vi "Argos_K_4.0 (SUPTNIK Customized Edition).vi"(0 "PID 1 COM":refnum<visa-resource-name>="COM1", 1 "Setpoint\n START":bool, 2 "Write to File":bool, 3 "SP 1 input (°C)":dbl=20.0 min=0.0 max=1300.0, 4 "Intervall (s)":u32=1 max=600, 5 "Write/\nRead":bool=TRUE, 6 "Delay (ms)":u32=500 min=100 max=600000, 7 "Auto Tune":bool, 9 "Standby":bool, 11 "Reset\nSTOPP":bool, 12 "ON":bool=TRUE caption="OFF", 13 "Get Values":bool, 15 "File Path":path) -> (8 "(°C)":dbl format="%#.3f", 14 "SP 1 is (°C)":dbl)   [LabVIEW 2013]
doc: "1. Verwendung\n\nDas Programm dient der Steuerung und Abfrage des Thermocontrollers I3252 und dem Auslesen von zwei VC 840 Messgeräten und einem Druckmessgerät Pfeiffer Single Gauge. \nDie Messgeräte werden Standardmäßig ausgelesen und erst nach Betätigung des Schalters \"Write to File\" in einer Textdatei abgespeichert. Das Eingabefeld \"Intervall\" legt den Abstand der Messpunkte fest.\nDer Setpoint für den Thermocontroller wird erst nach Betätigung des Tasters \"Setpoint START\" übernommen und angesteuert. Er wird ind den EEPROM des Gerätes geschrieben. Die Regelung kann mit Hilfe des Schalters \"Standby\" unterbrochen werden. Durch den Taster \"Reset STOPP\" kann der Setpoint aus dem EEPROM gelöscht werden.\nDie Eingabeflächen \"Constant\" und \"Thickness\" dienen der Berechnung des spezifischen Widerstands.\nDie Eingabeflächen \"User\" und \"Sample\" werden in den Header der Textdatei übernommen.\nDer Indikator \"File Path\" zeigt den aktuellen Speicherort der Textdatei an. Dieser wird nach ausschalten des Schalters \"Write to File\" gelöscht. Bei erneuten Schreiben muss ein neuer Speicherort gewählt werden. Bei Wahl desselben Speicherorts werden sämtliche bereits gespeicherte Daten gelöscht.\n\n\n2. Erläuterungen zum Blockdiagramm\n2.1 äußere Sequenz\nDie äußerte Sequenz besteht aus fünf Frames. Der erste dient der Initialisierung der Ports. Der zweite dient als Verzögerung um dem Programm genug Zeit zu geben die Ports zu öffnen. Jedoch senden die beiden VC 840 bereits Informationen an den Computer die in einem Puffer zwischengespeichert werden. Im dritten Frame wird dieser Puffer geleert. Somit kommt es zu keinem Framing Error. Desweiteren wird in diesem Frame die Startzeit der Messungen genommen. Im vierten Frame wird die eigentliche Messung und Verarbeitung der Daten durchgeführt. Die while-Schleife wird nur durch Auftreten eines Fehlers oder durch Betätigung des Stopbuttons auf dem Front Panel in der oberen linken Ecke unterbrochen. Im fünften und letzten Frame werden die Ports wieder geschlossen und beim Auftreten eines Fehlers wird das Programm automatisch gestoppt. Falls kein Fehler auftritt wird die Sequenz von vorne abgearbeitet.\n\n2.2 while-Schleife und innere Sequenz\n2.2.1 \"Event Structure\"\n2.2.1.1 Allgemein\nDer erste Frame beinhaltet ein \"Event Structure\". Dieser reagiert auf insgesamt elf verschiedene Ereignisse. Falls keines dieser Ereignisse auftreten sollte, warte die Struktur eine Millisekunde bevor die \"Event Structure\" verlassen wird. Die übrigen Ereignisse treten ein, wenn der entsprechende Kontroller eine Werteänderung erfährt.\n\n2.2.1.2 Event: Setpoint\nDieser Case besteht von außen nach innen aus einer Stacked Sequence, einer for-Loop und einer Flat Sequence die wiederum zwei \"Case Structures\" enthält. Als erstes wird bei dem Schalter \"Setpoint START\" der Blinkmodus aktiviert und bei dem Schalter \"Read Temperature\" deaktiviert. Danach folgt das eigentliche setzen des Temperatursollwerts. In der ersten Iteration wird dem Controller I3252 ein Schreibbefehl gesendet. Theoretisch kann der Setpoint in den RAM oder in den EEPROM geschrieben werden. Diese Auswahl erfolgt mit Hilfe des Schalters \"RAM\". Da das Schreiben in den RAM -Speicher aber aus diversen Gründen nicht erwünscht ist, wurde es nicht implementiert. Eine nachträgliche Implementierung ist aber leicht möglich, in dem die untere String-Konstante \"*P012\" durch \"*W012\" ersetzt wird. An diesem Befehl wird eine fünfstellige Hexadezimalzahl angehängt, die den Sollwert wiedergibt. Der Sollwert wird vorher mit zehn multipliziert, da das Komma standardmäßig nach der ersten Ziffer festgesetzt wurde (Bsp.: 800 wird gesendet um 80 einzustellen). Dieser Befehlsstrang wird an das Gerät mittels des SubVIs \"Comm_Interface\", auf welches später noch näher eingegangen wird, weitergegeben. Der durch das Gerät zurückgegebene String wird nicht verarbeitet.\nDie zweite Iteration dient dem Auslesen des eingestellten Sollwertes. Wahlweise kann der RAM- oder der EEPROM-Speicher ausgelesen werden. Die eigentliche Verarbeitung des Ausgabestrings erfolgt durch das SubVI \"Edit Setpoint\".\nDie Implementierung zur Einstellung des zweiten Setpoints erfolgt durch kopieren der ersten beiden Fälle und ersetzen der \"1\" im Befehf durch eine \"2\" (Bsp.: \"*P012\" zu \"*P022\"). Es darf aber nicht vergessen werden, dass dann ebenfalls die Anzahl der Iterationen angepasst werden muss.\nAls letztes wird der Blinkmodus des Schalters \"Setpoint START\" wieder deaktiviert.\n\n2.2.1.3 Event: Standby\nDieses Ereignis aktiviert bzw. deaktiviert als erstes den Blinckmodus des entsprechenden Schalters und sendet danach den Befehl zum aktivieren (\"*D03\") oder zum deaktivieren (\"*E03\") des Standbymodus an den Thermocontroller.\n\n2.2.1.4 Event: Set Command \nDer in das Feld \"Command shall be\" eingegebene Befehl wird an den Thermocontroller übermittlet. Die korrekte Form des Befehls ist im \"Communication Manuel\" nachzuschlagen. Das \"*\"-Zeichen wurde allerdings schon implementiert und muss somit nicht mit eingegeben werden.\n\n2.2.1.5 Event: Reset\nIn der ersten Iteration wird der Reset-Befehl an den Thermocontroller gesendet. In Folge wird der gesamte EEPROM-Speicher gelöscht. Deshalb wird in der zweiten Iteration der Setpoint aktualisiert. Dieser Befehl hat keinen Einfluss auf den RAM-Speicher. Die anschließende Wartezeit ist auf vier Sekunden festgesetzt und wurde empirisch ermittelt. Diese Zeit benötigt das Gerät um den Reset durchzuführen und für die Kommunikation wieder zur Verfügung zu stehen.\n\n2.2.1.6 Event: Auto Tune\nEs ist festgeschrieben, dass der Setpoint für die \"Auto Tune\"-Funktion wenigstens 20°C über der aktuellen Temperatur liegt. Deshalb wird zunächst der aktuelle Temperaturwert ausgelesen. Im zweiten Schritt werden zu diesem Wert zwanzig addiert und der Setpoint wird in den RAM-Speicher geschrieben. Das Schreiben in diesen Speicher ist nötig, da die \"Auto Tune\"-Funktion\" erst nach einem Reset startet. Im dritten Schritt wird der eigentliche Befehl für den \"Auto Tune\" gesendet (siehe dazu \"Communication Manuel\" S.27). Als vierte und letzte Iteration der for-Schleife folgt der bereits erwähnte Reset-Befehl. Der Temperatursollwert, der im RAM-Speicher eingetragen ist, muss zum Schluss wieder auf 0°C gesetzt werden. Die Zeit für die Ausführung des \"Auto Tune\"-Befehls wurde empirisch ermittelt und 45 s festgesetzt.\n\n2.2.1.7 Event: Write LOW/HI\nDieses Ereignis setzt die am Analogausgang anliegende Spannung fest. Normalerweise beträgt dieser Spannungswert 0-10 V. Das angeschlossene Netzteil verträgt aber maximal nur 2,3 V. Aus diesem Grund wird der \"%HIGH\" auf 23 gesetzt. Somit beträgt die maximal anliegende Spannung nur noch 23% von der maximal möglichen, d.h 2,3V. Ein niedrigerer Wert ist jederzeit möglich, genauso wie ein höherer für den Parameter \"%LOW\". Diese werden zunächst nacheinander in den RAM-Speicher geschrieben und anschließend wieder ausgelesen.\n\n2.2.1.8 Event: Set PID\nDie Werte für den PID-Regler können sowohl mit Hilfe der \"Auto Tune\"-Funktion, als auch manuell eingestellt werden. Es wird wiederum zwischen dem Schreiben in den RAM- und dem EEPROM-Speicher unterschieden. Zunächst werden die Werte für \"P\", \"I\" und \"D\", in dieser Reihenfolge, gesetzt und danach die aktuellen Werte ausgelesen.\n\n2.2.1.9 Event: Get Values\nDieses Ereignis hat zur Folge, dass die Werte für \"P\", \"I\", \"D\", \"%LOW\", \"%HIGH\" und des Setpoints wahlweise aus dem RAM- oder EEPROM-Speicher gelesen werden. Die aktuellen Werte werden nicht nur in die entsprechenden Anzeigefelder übernommen, sondern auch in die entsprechenden Eingabefelder, mit Ausnahme des Temperatursollwerts. \n\n2.2.1.10 Event: RAM\nPrinzipiell kann zwischen dem Schreiben in den RAM- oder EEPROM-Speicher des Thermocontrollers gewählt werden. Die entsprechende Schalterposition auf dem Frontpanel zeigt den aktuell verwendeten Speicher an. Die Anzeigewerte werden bei jedem Umschalten aktualisiert und sind im entsprechenden Speicher eingetragen. Die Implementierung ist identisch mit der des Ereignisses \"Get Values\". Es gilt zu beachten, dass die Werte für \"%LOW\" und \"%HIGH\" nur in den RAM-Speicher geschrieben werden können und somit auch nur aus diesem ausgelesen werden können.\n\n2.2.1.11 Event: Set Gauge to Zero\nMit Hilfe der SubVIs \"Get Pressure\" und \"Offset Display\" werden die Werte für den alten und den neuen Offset und der durch den zweiten Drucksensor ermittelt Druck ermittelt. \n\n2.2.1.12 Event: Write to File\nSollte der Schalter \"Write to File\" aktiviert werden, d.h. Schalterposition oben, so wird zunächst durch das SubVI \"Header\" ein Header für die unter \"File Path\" definierte Datei angelegt. Alle Werte, die bereits in der entsprechenden Datei stehen, werden dabei gelöscht.\n\n2.2.2 \"Timed Structures\"\nIm dritten Frame der inneren Sequenz werden die Werte für Zeitpunkt, Temperatur, Spannung, Strom und Druck ermittelt. Damit die Werte zum gleichen Zeitpunkt aufgenommen werden, werden \"Timed Sequences\" eingesetzt. Mit dem entsprechenden Schalter auf dem Front Panel unter dem Tab \"Settings\" kann gewählt werden, ob das entsprechende Gerät ausgelesen werden soll oder nicht. Die einzelnen Sequenzen werden parallel abgearbeitet, womit die Prozesszeit von diesem Frame durch der zeitintensivsten Sequenz abhängt. Dies ist in aller Regel das Auslesen der Temperatur, da ein \"Delay\" von 500 ms oder größer benötigt wird, um den Controller ordentlich ansprechen zu können.\nDie Systemzeit wird durch das SubVI \"System Time in Seconds\" in Sekunden umgerechnet und der in dem Parameter \"Starttime\" gespeicherte Wert wird abgezogen. Somit werden die Sekunden seit dem Start des Programms gezählt.\n\n2.2.3 restlichen Frames\nIm zweiten Frame wird das Intervall zwischen den einzelnen Messwerten festgelegt. Dabei wird der Wert des Parameters \"Delay\" abgezogen. Dieser Wert beträgt im Normalfall 500 ms und ist somit nicht vernachlääsigbar.\nDer Vierte Frame beinhaltet die Umrechnung des Temperatur-Strings in einen Temperaturwert durch das SubVI \"Edit Tmperature\", die Berechnung des spezifischen Widerstands durch das SubVI \"Resistivity Calculation\" und die Überprüfung des Druckwerts. Auch werden die neu gewonnen Werte in das entsprechende Shift-Register übernommen. Falls der Druckwert einen in dem Parameter \"Pressure Limit (mbar)\" festgelegten Grenzwert überschreiten sollte, wird der Thermocontroller automatisch in den Standby-Modus versetzt. Des Weiteren wird der Schalter \"Standby\" solange gesperrt, wie der Druck oberhalb des Grenzwertes liegt. Wenn der Druck wieder unter den Grenzwert gesunken ist, wird der Standby-Befehl nicht automatisch aufgehoben, sondern muss vom Benutzer durch Betätigung des entsprechenden Schalters gegeben werden.\nIm fünften Frame werden die Diagramme erstellt. Dabei wird jedes Mal von neuem das gesamte Shift-Register als Graph dargestellt. Weiterhin werden die Messwerte in ein 1D-Array geschrieben.\nDer sechste und letzte Frame beinhaltet den eigentlich Schreibvorgang der Messwerte in eine Textdatei und die Überprüfung ob ein Fehler vorliegt.\n\n2.3 SubVIs\n2.3.1 Allgemein\nDie SubVIs für die Messgeräte VC840 und das Druckmessgerät wurden aus anderen Quellen übernommen. \n\n2.3.2 \"Header\"\nIn den Header wird zunächst das aktuelle Datum und die aktuelle Zeit übernommen. Die ausgewählte Datei wird dabei überschrieben. Danach wird der Name des Benutzers und der Probe übernommen. Zum Schluss werden die Einheiten in einer Reihe, durch einen Tabulator getrennt, in den Header geschrieben.\n\n2.3.3 \"I3252 Comm Interface\"\nDieses VI stellt die Kommunikation mit dem Thermocontroller her und gibt den Ausgabe-String zurück.\n\n2.3.4 \"I3252 Edit Setpoint\"\nIm Ausgabe-String vom Thermocontroller ist an der vierten Stelle die Stelle des Dezimalpunktes verschlüsselt. Dieses Hexadezimalzahl wird herausgefiltert und an ein \"ENUM Controller\" übergeben. Dieser weist der Hexadezimalzahl eine Nummer zu, mit welcher ein Wert aus einem Array entnommen wird. Dieser Wert dient als Quotient. Der tatsächliche Wert kann somit errechnet werden.\n\n2.3.5 \"I3252 Edit Temperature\"\nDer Temperatur-String, der vom Thermocontroller zurückgegeben wird, wird in eine Dezimalzahl umgewandelt. Manchmal kommt es aus zu Dropouts, die durch dieses Programm herausgefiltert werden. Der letzte Wert wird dabei in einer \"Feedback Node\" gehalten unter der Annahme, dass sich der Temperaturwert nicht sprunghaft ändert.\n\n2.3.6 \"Resistivity Calculation\"\nDer spezifische Widerstand wird nach folgender Formel ausgerechnet. Dabei entspricht t der Dicke der Probe und C ist eine Konstante.\nrho=C*pi*t*U/(ln( 2)*I)\n\n2.3.7 \"System Time in Seconds\"\nZunächst wird die aktuelle Systemzeit ausgelesen. Danach wird diese in Stunden, Minuten und Sekunden aufgeteilt, alles in Sekunden umgerechnet und letztendlich addiert."
uses:
  <vilib>/Platform/TimedLoop/XDataNode/timing_clust.ctl
  <vilib>/Platform/TimedLoop/XDataNode/nitl_modes.ctl
  <vilib>/Platform/TimedLoop/XDataNode/wakeup.ctl
  <vilib>/Instr/_visa.llb/VISA Configure Serial Port (Instr).vi
  <vilib>/Platform/TimedLoop/scheduler/LVUserAPI/_suppVIs/Create_1kHz_TSource.vi
  <vilib>/Utility/file.llb/Write To Spreadsheet File (DBL).vi
  <vilib>/Platform/TimedLoop/XDataNode/XDataNode.xnode
  <vilib>/Platform/TimedLoop/XDataNode/XDNodeRunTimeDep.lvlib
  Argos0v7/Dependencies/Pfeiffer TPG261+262 Single+Dual Gauge/Dual Gauge.lvlib
panel:
  out "appended array":dbl[](array[numeric])
  in  "Tab Control":T1(tab)
  out "Get Actual Set Point":dbl
  in  "Get SetPoint":bool
  in  "Setpoint":dbl=10.0
  in  "Minutes":dbl
  in  "Hours":dbl
  in  "Soak Minutes":dbl=1.0
  in  "Soak Hours":dbl
  in  "Ramp":bool
  in  "Sample":string
  in  "User":string
  out "Thermocouple (Sample holder 1)":cluster{dbl[], dbl[]}(graph)
  out "current time (s)":dbl
  out "data logger intervall (s)":dbl
  out "loop time (s)":dbl
  in  "stop":bool
  out "TPG 1":cluster{dbl[], dbl[]}[](graph)
  out "Pressure Baratron 2":dbl format="%#_4e"
  out "Pressure FullRange 2":dbl format="%#_3e"
  out "Pressure OpenPort":cluster{dbl[], dbl[]}(graph)
  out "Pressure OpenPort2":dbl caption="current"
  in  "PID 2 COM":refnum<visa-resource-name>="COM8"
  in  "Baud Rate 2":u32=9600
  in  "Data Bits 2":u16=7 min=5 max=8 step=1
  in  "Parity 2":u16(ring)=1 items=["None", "Odd", "Even", "Mark", "Space"]
  in  "Stop Bits 2":u16(ring)=10 items=["1.0"=10, "1.5"=15, "2.0"=20]
  in  "Flow Control 2":u16(ring) items=["None"=0, "XON/XOFF"=1, "RTS/CTS"=2, "DTR/DSR"=4]
  in  "Delay (ms) 2":u32=500 min=100 max=600000
  in  "Write/\nRead 2":bool=TRUE
  out "status 2":bool caption="Status"
  out "code 2":i32 caption="Code"
  out "code":i32 caption="Code"
  out "status":bool caption="Status"
  in  "Set Gauge to Zero":bool
  out "Status Gauge 1#2":i32(ring) items=["data OK", "underrange", "overrange", "sensor error", "sensor off", "no sensor", "ID error"]
  out "Pressure Gauge 1#2":dbl format="%.3e"
  out "Pressure Gauge 1#1":dbl format="%.3e"
  out "Status Gauge 1#1":i32(ring) items=["data OK", "underrange", "overrange", "sensor error", "sensor off", "no sensor", "ID error"]
  in  "TPG 1 COM":refnum<visa-resource-name>="COM5"
  in  "Pressure Limit (mbar)":dbl=1.0 min=0.0 max=1100.0
  out "Current Offset (mbar)":dbl
  in  "ON (TPG 2)":bool caption="OFF"
  in  "ON (TPG 1)":bool=TRUE caption="OFF"
  in  "ON":bool caption="OFF"
  in  "VC 840 2":refnum<visa-resource-name>="COM8"
  out "Reading 2":dbl format="%_4f"
  out "Mode 2":enum16{"?", "Diode", "Beep", "DC", "AC"}(ring)
  out "Unit 2":string
  in  "VC 840 1":refnum<visa-resource-name>="COM8"
  out "Reading 1":dbl format="%_4f"
  out "Mode 1":enum16{"?", "Diode", "Beep", "DC", "AC"}(ring)
  out "Unit 1":string
  out "Status 1":T2
  out "Status 2":T2
  in  "ON":bool caption="OFF"
  out "% HIGH Istwert":u32
  out "% LOW Istwert":u32
  in  "% High Sollwert":u32=23 max=24
  in  "% LOW Sollwert":u32 max=25
  in  "RAM":bool=TRUE caption="EEPROM"
  out "D (Rate) IstWert":u32
  out "I ( Reset1) Istwert":u32
  out "P (PB1) Istwert":u32 caption="actual value"
  in  "D (Rate) Sollwert":u32 max=3999
  in  "I ( Reset1) Sollwert":u32 max=3999
  in  "P (PB1) Sollwert":u32 caption="set value" max=9999
  in  "Set Command":bool
  in  "Set PID":bool
  in  "Write LOW/HI":bool
  in  "Flow Control":u16(ring) items=["None"=0, "XON/XOFF"=1, "RTS/CTS"=2, "DTR/DSR"=4]
  in  "Stop Bits":u16(ring)=10 items=["1.0"=10, "1.5"=15, "2.0"=20]
  in  "Parity":u16(ring)=1 items=["None", "Odd", "Even", "Mark", "Space"]
  in  "Data Bits":u16=7 min=5 max=8 step=1
  in  "Baud Rate":u32=9600
  out "Command output":string
  in  "Command input":string
  in  "TPG 2 COM":refnum<visa-resource-name>="COM8"
  out "Pressure Gauge 2#2":dbl format="%.3e"
  out "Pressure Gauge 2#1":dbl format="%.3e"
  out "Status Gauge 2#2":i32(ring) items=["data OK", "underrange", "overrange", "sensor error", "sensor off", "no sensor", "ID error"]
  out "Status Gauge 2#1":i32(ring) items=["data OK", "underrange", "overrange", "sensor error", "sensor off", "no sensor", "ID error"]
  out "Current":cluster{dbl[], dbl[]}(graph)
  out "Voltage":cluster{dbl[], dbl[]}(graph)
  out "Voltage (V)":dbl format="%.4e"
  out "Current (A)":dbl format="%.4e"
  out "Resistivity":cluster{dbl[], dbl[]}(graph)
  out "Resistivity (Ohm*cm)":dbl format="%.3e"
  out "Pirani (VVP1 Scroll)":cluster{dbl[], dbl[]}(graph)
  in  "4PP constant":dbl min=0.0 max=5.0
  in  "Thickness (nm)":dbl min=0.0
  out "Pressure Pirani 2":dbl format="%#_3e"
  # "set \nvalue"
  # "actual \nvalue"
  # "T (°C)"
  # "Ramp And Soak Toolkit"
  # "Ramp"
  # "Soak"
  # "mbar"
  # "mbar"
  # "mbar"
  # "Pressure Measurement \n(Pfeiffer TPG261)"
  # "PID Controller (Omega Newport i3252)"
  # "PID Controller (Omega Newport i3252)"
  # "limit (mbar)"
  # "Multimeter\n#1 (VC 840)"
  # "Multimeter\n#2 (VC 840)"
  # "P"
  # "I"
  # "D"
  # "% Low"
  # "% High"
  # "mbar"
  # "Authors:  Daniel Schuster (sir-dan@web.de)\n                 Steffen Cornelius (s.cornelius@hzdr.de)\n                 Nico Spahn (x)\n\n                 premade SubVIs for readout of Pfeiffer gauge and VC840 Multimeters were used\n                 SubVI \"I3252_Comm_Interface\" is based on a modified Labview example\n\nRelease:  v1.0    \n\nVersion History:\n\nv1.1  -    28.06.2011\n             - Format des Files geändert von %.3f auf %g\n             - maximale Eingabewerte für PID begrenzt\nv1.2  -    12.07.2011\n             - Anzeige p,rho, U, V auf Scientific geändert\n             - y-Achse p,rho auf Log geändert\n             - numerische Zeitanzeige hinzugefügt\n             - 4PP Constant: pi/ln(2)=4,532 set as the default value\nv1.3  -    25.07.2011\n             - Zeitvariable auf EXT geändert, um Sprünge in Diagrammen loszuwerden\nv1.4  -   27.07.2011\n             - ALLE Variablen auf DBL zurückgesetzt wegen Formatierungsproblem im File\n             - Zeitberechnung neu gemacht (Tick count differenzen) -> Zeitsprünge korrigiert ?\n             - Delay/Intervall überarbeitet\nv1.5  -   05.12.2012\n                - Austausch der alten Pfeifer SubvIs durch neue -> nun alle 4 Kanäle des DualGauge\n                                                                                                         Controllers gleichzeitig auslesbar\n                - neue Pfeiffer SubVIs verwendet in Druckwertauslesung und Offset Berechnung des Baratron\n                  Druckes (COM5 Sensor1)\n                - Neuarragement des GUI -> FullRange und Baratron neben Temperatur auf Haupseite zu sehen\n                                                                   Pirani und OpenPort auf Meas.2 zu sehen\n                                                                   Diagnose Seite umfasst nun auch Widerstandsdiagramm\n                - Änderungen der Settingseite -> nun alle 4 Drucksensoren mit aktuellem Messwert und Gerätestatus\n                                                                           zu sehen\n                - The readout of the PID-Temperature Controller and the VC840 Multimeters was not modified\nv1.73  -  18.10.2013\n                - Layout Änderungen\nv.1.8   -  19.01.2014\n                - Änderung Layout Settings Tab\n                - Trennung der beiden TPG Dual Gauge Controls\n                -"
  # "Version 1.73    - last change 18.10.2013"
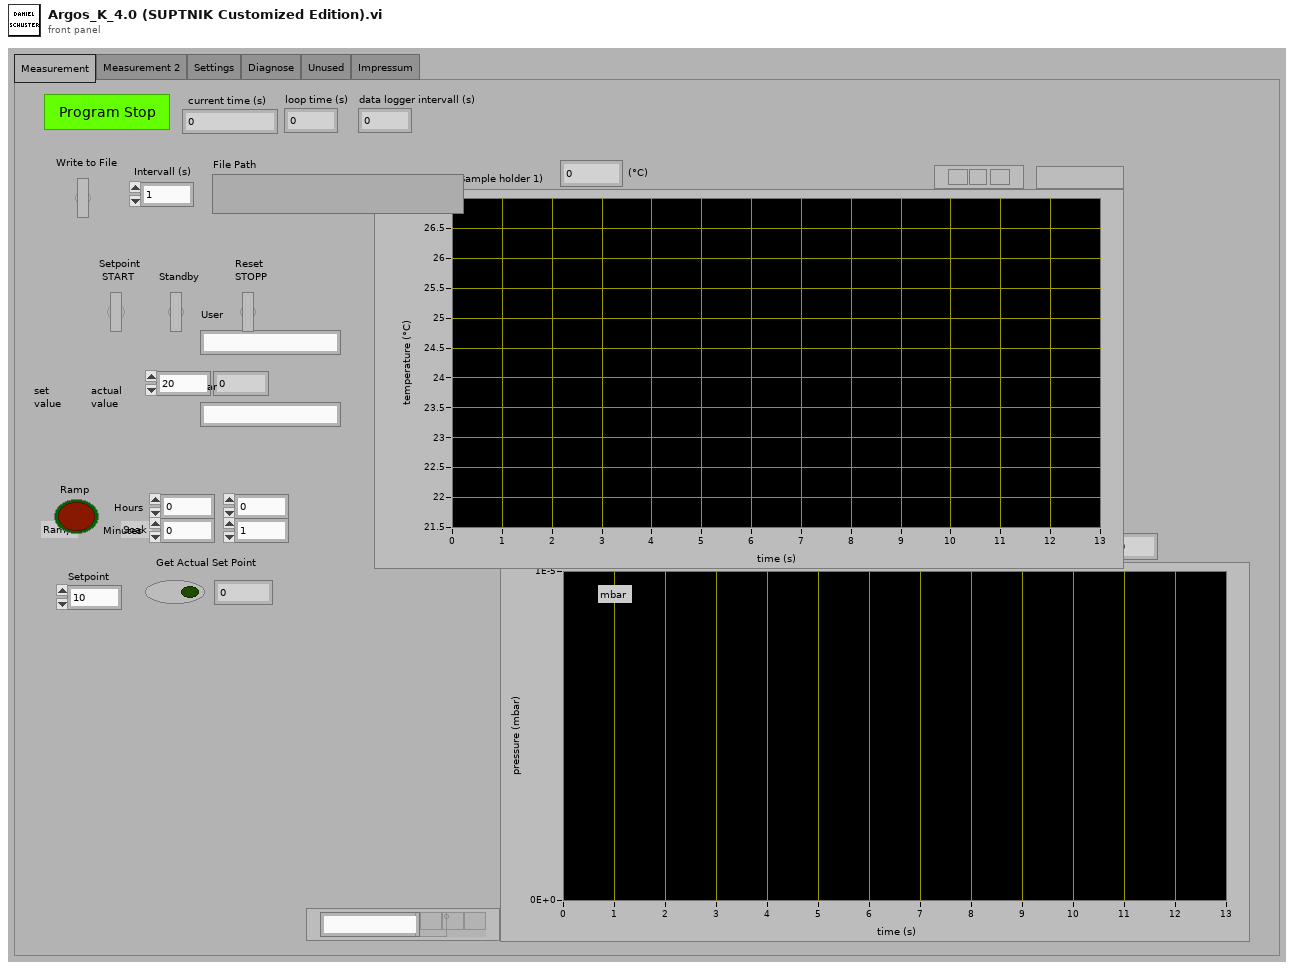
[diagram p1: front panel]
types:
  T1 = enum32{"Measurement", "Measurement 2", "Settings", "Diagnose", "Unused", "Impressum"}
  T2 = cluster{"Low Bat":bool, "Auto":bool, "Delta":bool, "Hold":bool, "RS232":bool}
  T3 = typedef "XDNodeRunTimeDep.lvlib/timing_clust.ctl" = cluster{"Expected End [f-1]":u64, "Actual End [f-1]":u64, "Finished Late? [f-1]":bool, "Expected End [i-1]":u64, "Actual End [i-1]":u64, "Finished Late? [i-1]":bool, "Expected Start [i]":u64, "Actual Start [i]":u64, "Expected Start [f]":u64, "Actual Start [f]":u64, "Source Name":string, "Structure Name":string, "Period":i64, "Deadline":i64, "Offset":i64, "Start":i64, "Priority":i32, "Timeout":i32, "Mode":T4, "Wakeup Reason":T5, "Error":errorcluster, "Source Type":string, "Secondary Source Type":string, "Global End Time":u64, "Global Start Time":u64, "Frame Duration":u64, "Iteration Duration":u64, "Assigned CPU":i32, "I/O Scan Engine Mode":u32}
  T4 = typedef "XDNodeRunTimeDep.lvlib/nitl_modes.ctl" = enum32{"No Change", "Process missed periods, maintain original phase", "Discard missed periods, maintain original phase", "Process missed periods, ignore original phase", "Discard missed periods, ignore original phase"}
  T5 = typedef "XDNodeRunTimeDep.lvlib/wakeup.ctl" = enum32{"Normal", "Aborted", "Asynchronous wakeup", "Timing source error", "Timed loop error", "Timeout"}
  T6 = enum8{"Enabled", "Disabled", "Disabled and Grayed Out"}
  T7 = cluster{"VISA resource name out":refnum<visa-resource-name>, "error out":errorcluster, "Delay (ms)":u32, "Write/\nRead":bool}
  T8 = cluster{"VISA resource name out":refnum<visa-resource-name>, "error out":errorcluster, "Delay (ms) 2":u32, "Write/\nRead 2":bool}
  T9 = cluster{"TPG 2 COM":refnum<visa-resource-name>, "error out":errorcluster}
  T10 = cluster{"COM out":refnum<visa-resource-name>, "Cluster (Ausgang)":errorcluster}
  T11 = cluster{"Pressure Gauge#1":dbl, "Pressure Gauge#2":dbl}
  T12 = cluster{"TPG 1 COM":refnum<visa-resource-name>, "error out":errorcluster}
  T13 = cluster{"COM out":refnum<visa-resource-name>, "error out":errorcluster, "COM out":refnum<visa-resource-name>, "error out":errorcluster}
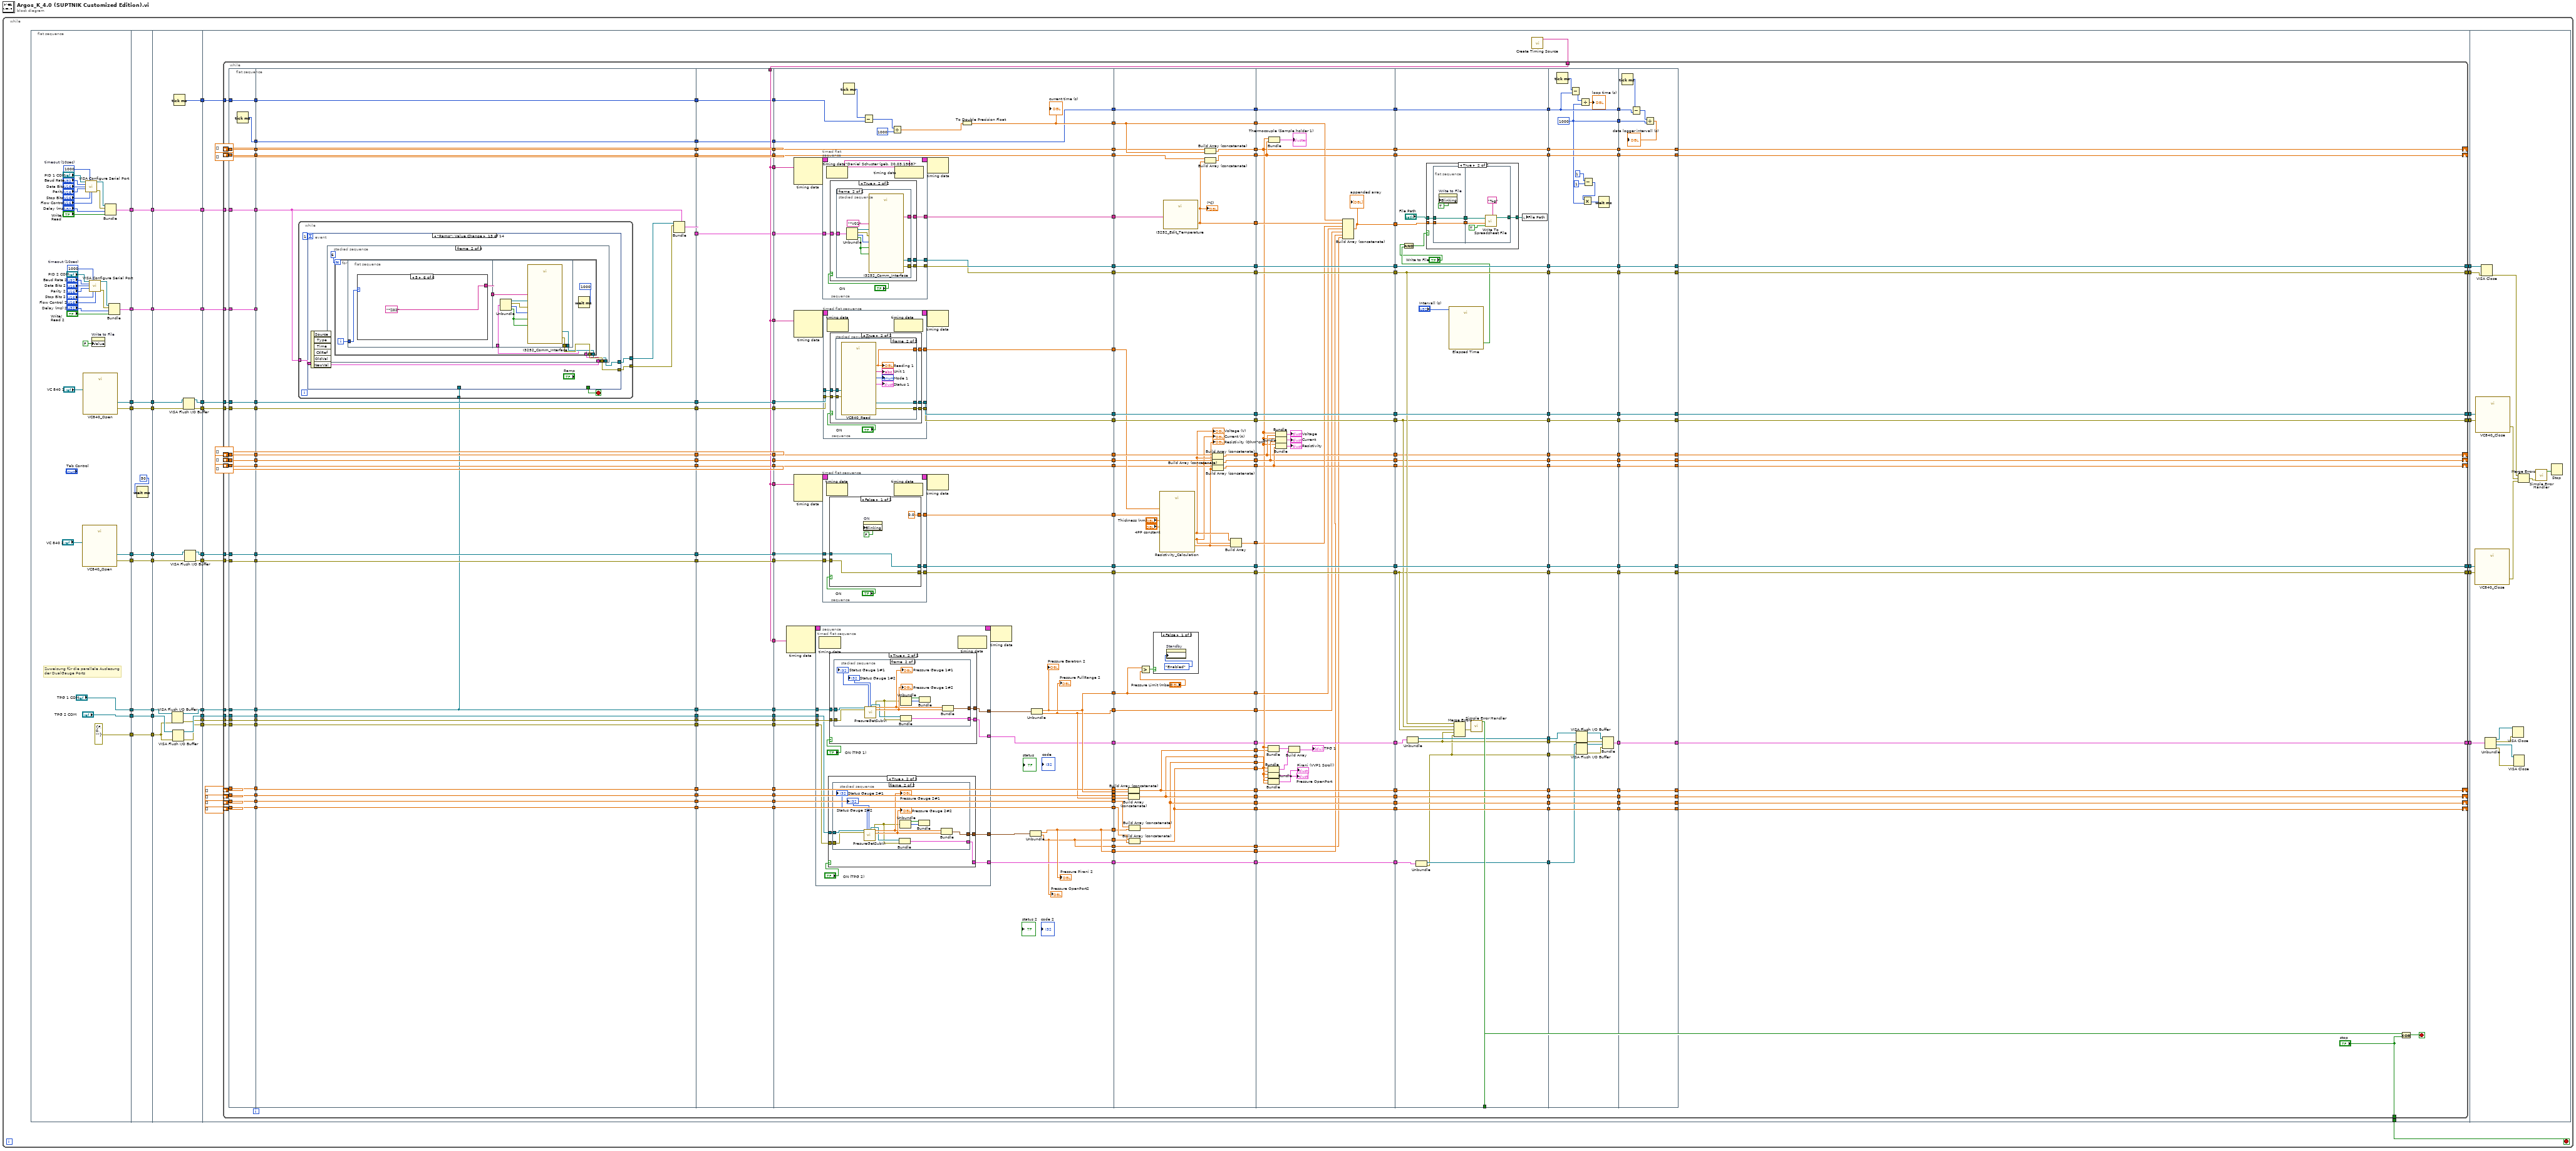
[diagram p0: block diagram]
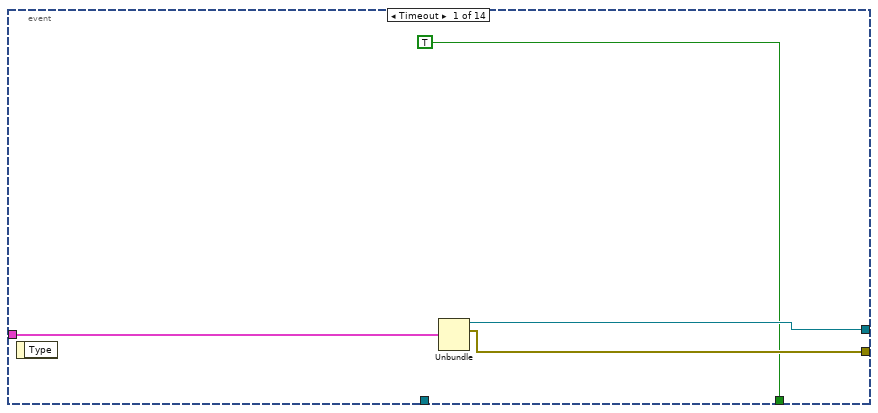
[diagram p2: hidden frame]
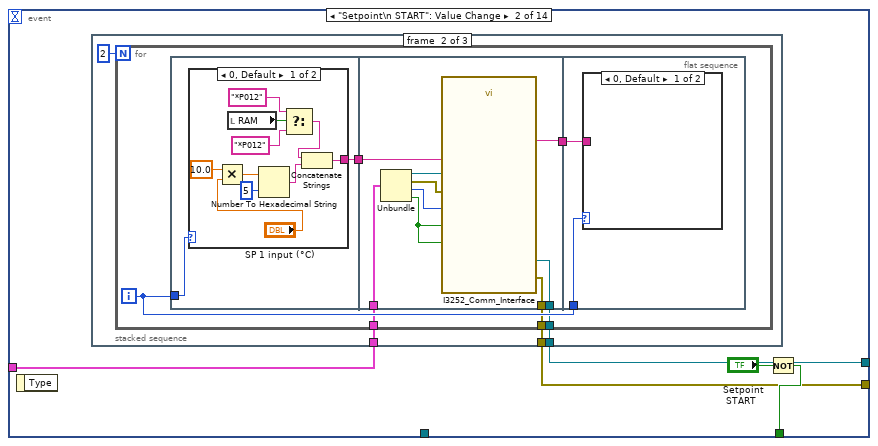
[diagram p3: hidden frame]
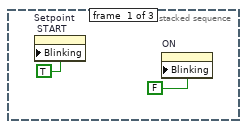
[diagram p4: hidden frame]
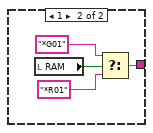
[diagram p5: hidden frame]
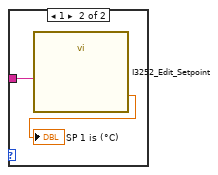
[diagram p6: hidden frame]
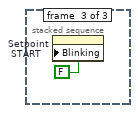
[diagram p7: hidden frame]
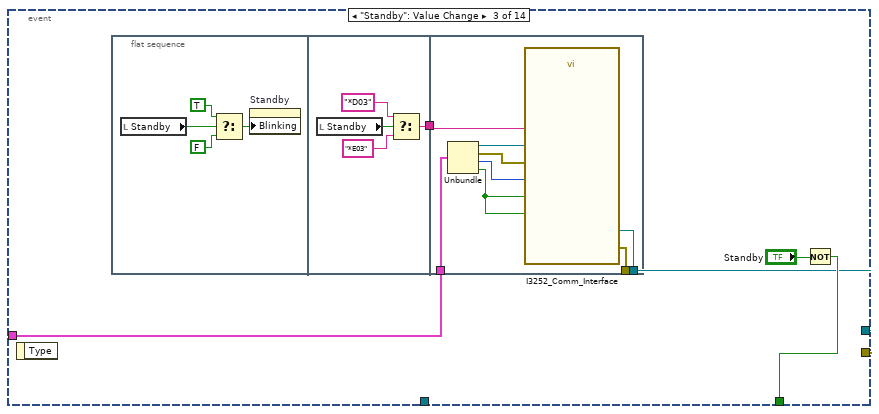
[diagram p8: hidden frame]
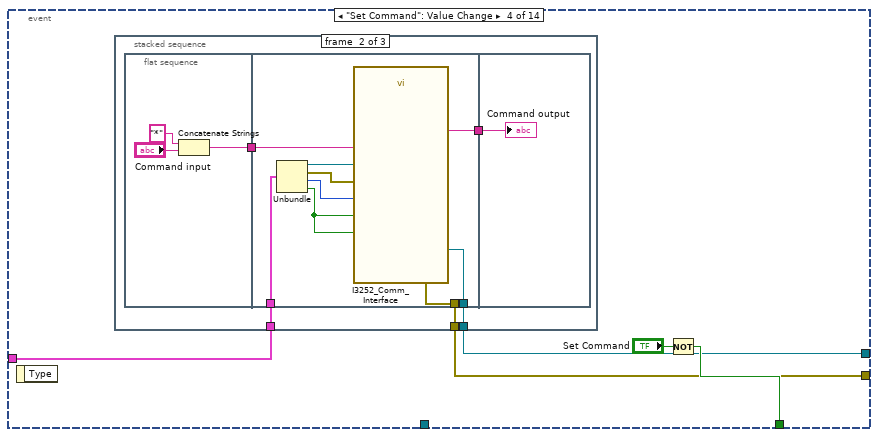
[diagram p9: hidden frame]
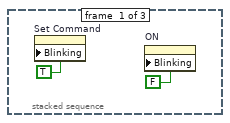
[diagram p10: hidden frame]
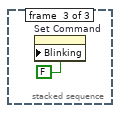
[diagram p11: hidden frame]
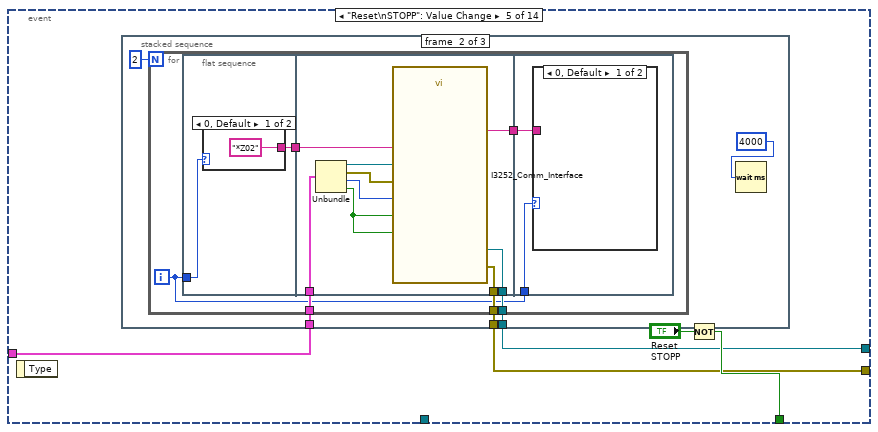
[diagram p12: hidden frame]
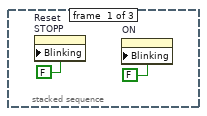
[diagram p13: hidden frame]
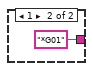
[diagram p14: hidden frame]
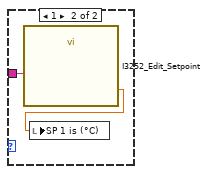
[diagram p15: hidden frame]
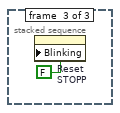
[diagram p16: hidden frame]
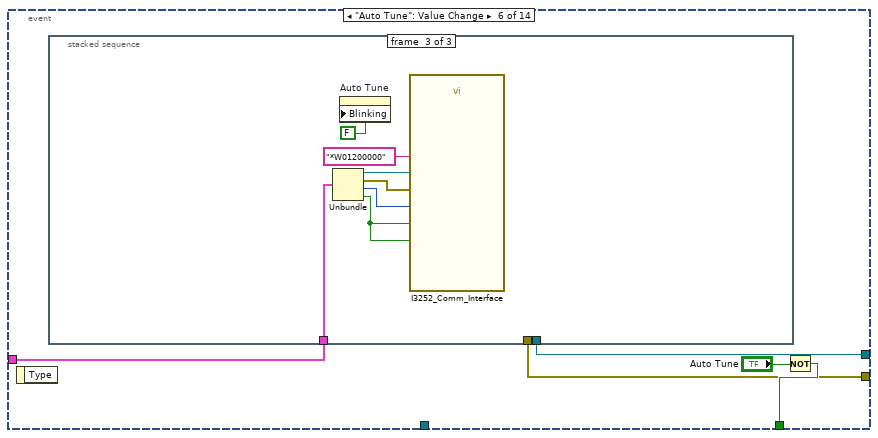
[diagram p17: hidden frame]
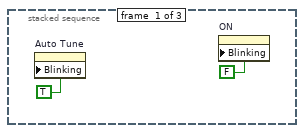
[diagram p18: hidden frame]
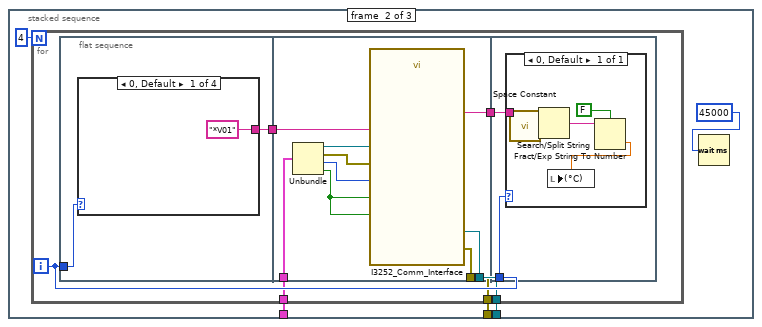
[diagram p19: hidden frame]
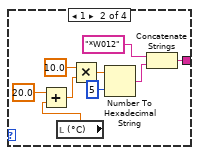
[diagram p20: hidden frame]
diagram:
  n1 = while {
    stop <- w9 stop-if-true
    n2 = flat-sequence {
      tunnel: [w70] -> w37
      tunnel: [w71] -> w36
      tunnel: [w56] -> w35
      tunnel: [w69] -> w34
      tunnel: [w68] -> w33
      tunnel: ["TPG 1 COM"] -> w32
      tunnel: ["TPG 2 COM"] -> w31
      tunnel: [errorcluster {"status"=FALSE, "code"=0, "source"=""} ("Fehler (Eingang)")] -> w6
      tunnel: [w39] -> w1
      tunnel: w37 -> [w81]
      tunnel: [w81] -> w30
      tunnel: w36 -> [w80]
      tunnel: [w80] -> w29
      tunnel: w35 -> [w79]
      tunnel: [w79] -> w28
      tunnel: w34 -> [w78]
      tunnel: [w78] -> w27
      tunnel: w33 -> [w77]
      tunnel: [w77] -> w26
      tunnel: [w75] -> w25
      tunnel: w32 -> [w75]
      tunnel: [w74] -> w24
      tunnel: w31 -> [w74]
      tunnel: [w73] -> w7
      tunnel: w6 -> [w73]
      tunnel: [w72] -> w2
      tunnel: w1 -> [w72]
      tunnel: w30 -> [w93]
      tunnel: [w92] -> w23
      tunnel: w29 -> [w94]
      tunnel: [w91] -> w22
      tunnel: w28 -> [w99]
      tunnel: [w99] -> w21
      tunnel: w27 -> [w96]
      tunnel: [w97] -> w20
      tunnel: w26 -> [w95]
      tunnel: [w98] -> w19
      tunnel: [w90] -> w18
      tunnel: [w88] -> w17
      tunnel: w25 -> [w89]
      tunnel: [w87] -> w16
      tunnel: w24 -> [w86]
      tunnel: w7 -> [w85]
      tunnel: [w84] -> w5
      tunnel: [w83] -> w4
      tunnel: [w82] -> w3
      tunnel: w2 -> [w82]
      tunnel: w23 -> [w128]
      tunnel: w22 -> [w127]
      tunnel: w21 -> [w126]
      tunnel: w20 -> [w124]
      tunnel: w19 -> [w123]
      tunnel: [w122] -> w15
      tunnel: [w121] -> w14
      tunnel: [w120] -> w13
      tunnel: [w119] -> w12
      tunnel: [w118] -> w11
      tunnel: [w117] -> w10
      tunnel: w18 -> [w111]
      tunnel: w17 -> [w110]
      tunnel: w16 -> [w109]
      tunnel: [w104] -> w9
      tunnel: [w103] -> w8
      tunnel: w5 -> [w102]
      tunnel: w4 -> [w101]
      tunnel: w3 -> [w100]
      tunnel: w15 -> [w1425]
      tunnel: w14 -> [w1424]
      tunnel: w13 -> [w1427]
      tunnel: w12 -> [w1426]
      tunnel: w11 -> [w1429]
      tunnel: w10 -> [w1428]
      tunnel: w8 -> [w1422]
      frame #0 {
        w40 = u32 1000  # timeout (10sec)
        w57 = u32 1000  # timeout (10sec)
        # "Zuweisung für die parallele Auslesung\nder DualGauge Ports"
        n3 = call "VC840_Open.vi"("VISA resource name"="VC 840 2") -> ("error out"=w68:errorcluster, "VISA resource name out"=w69:refnum<visa-resource-name>)  [unwired: 1 in, 8 out]
        n4 = call "VC840_Open.vi"("VISA resource name"="VC 840 1") -> ("error out"=w71:errorcluster, "VISA resource name out"=w70:refnum<visa-resource-name>)  [unwired: 1 in, 8 out]
        n5 = call-poly "VISA Configure Serial Port"("VISA resource name"="PID 1 COM", "timeout (10sec)"=w57, "baud rate (9600)"="Baud Rate", "data bits (8)"="Data Bits", "parity (0:none)"="Parity", "stop bits (10: 1 bit)"="Stop Bits", "flow control (0:none)"="Flow Control") -> ("VISA resource name out"=w66:refnum<visa-resource-name>, "error out"=w67:errorcluster)  [unwired: 2 in, 5 out]
        n6 = call-poly "VISA Configure Serial Port"("VISA resource name"="PID 2 COM", "timeout (10sec)"=w40, "baud rate (9600)"="Baud Rate 2", "data bits (8)"="Data Bits 2", "parity (0:none)"="Parity 2", "stop bits (10: 1 bit)"="Stop Bits 2", "flow control (0:none)"="Flow Control 2") -> ("VISA resource name out"=w49:refnum<visa-resource-name>, "error out"=w50:errorcluster)  [unwired: 2 in, 5 out]
        n7 = property on="Write to File" class="Bool (strict)"("Value"=FALSE ("Write to File")) -> ()  [unwired: 2 in, 2 out]
        n8 = Bundle("VISA resource name out"=w66, "error out"=w67, "Delay (ms)"="Delay (ms)", "Write/\nRead"="Write/\nRead") -> (w56:T7)  [unwired: 1 in]
        n9 = Bundle("VISA resource name out"=w49, "error out"=w50, "Delay (ms) 2"="Delay (ms) 2", "Write/\nRead 2"="Write/\nRead 2") -> (w39:T8)  [unwired: 1 in]
      }
      frame #1 {
        n10 = Wait (ms)(milliseconds to wait=u32 50) -> ()  [unwired: 1 out]
      }
      frame #2 {
        n11 = VISA Flush I/O Buffer(VISA resource name=w89, error in (no error)=w85) -> (VISA resource name out=w88:refnum<visa-resource-name>, error out=w84:errorcluster)  [unwired: 1 in]
        n12 = VISA Flush I/O Buffer(VISA resource name=w86, error in (no error)=w85) -> (VISA resource name out=w87:refnum<visa-resource-name>, error out=w83:errorcluster)  [unwired: 1 in]
        n13 = Tick Count (ms)() -> (millisecond timer value=w90:u32)
        n14 = VISA Flush I/O Buffer(VISA resource name=w93, error in (no error)=w94) -> (VISA resource name out=w92:refnum<visa-resource-name>, error out=w91:errorcluster)  [unwired: 1 in]
        n15 = VISA Flush I/O Buffer(VISA resource name=w96, error in (no error)=w95) -> (VISA resource name out=w97:refnum<visa-resource-name>, error out=w98:errorcluster)  [unwired: 1 in]
      }
      frame #3 {
        n16 = call-poly <vilib>:"Create Timing Source.vi"() -> ("name (out)"=w125:string)  [unwired: 10 in, 1 out]
        n17 = while {
          tunnel: w128 -> [w349]
          tunnel: w127 -> [w348]
          tunnel: w126 -> [w347]
          tunnel: w125 -> [w340]
          tunnel: w124 -> [w333]
          tunnel: w123 -> [w332]
          tunnel: [w328] -> w122
          tunnel: [w327] -> w121
          tunnel: [w325] -> w120
          tunnel: [w323] -> w119
          tunnel: [w321] -> w118
          tunnel: [w319] -> w117
          shift-right: [w292] -> _
          shift-left: dbl[] [] -> [w297]
          shift-right: [w270] -> _
          shift-left: dbl[] [] -> [w305]
          shift-right: [w294] -> _
          shift-left: dbl[] [] -> [w301]
          shift-right: [w267] -> _
          shift-left: dbl[] [] -> [w304]
          shift-right: [w264] -> _
          shift-left: dbl[] [] -> [w303]
          tunnel: w111 -> [w258]
          tunnel: w110 -> [w214]
          tunnel: w109 -> [w210]
          shift-right: [w168] -> _
          shift-left: dbl[] [] -> [w198]
          shift-right: [w166] -> _
          shift-left: dbl[] [] -> [w196]
          shift-right: [w164] -> _
          shift-left: dbl[] [] -> [w194]
          shift-right: [w162] -> _
          shift-left: dbl[] [] -> [w192]
          tunnel: ["stop"] -> w104
          tunnel: [w156] -> w103
          tunnel: w102 -> [w151]
          tunnel: w101 -> [w149]
          tunnel: w100 -> [w129]
          stop <- w155 stop-if-true
          n18 = flat-sequence {
            tunnel: w258 -> [w360]
            tunnel: w297 -> [w361]
            tunnel: w301 -> [w362]
            tunnel: w303 -> [w363]
            tunnel: w304 -> [w364]
            tunnel: w305 -> [w365]
            tunnel: w332 -> [w366]
            tunnel: w333 -> [w367]
            tunnel: w347 -> [w368]
            tunnel: w348 -> [w369]
            tunnel: w349 -> [w370]
            tunnel: [w370] -> w257
            tunnel: [w369] -> w256
            tunnel: [w368] -> w255
            tunnel: [w367] -> w254
            tunnel: [w366] -> w253
            tunnel: [w365] -> w252
            tunnel: [w364] -> w251
            tunnel: [w363] -> w250
            tunnel: [w362] -> w249
            tunnel: [w361] -> w248
            tunnel: [w360] -> w247
            tunnel: [w359] -> w229
            tunnel: [w358] -> w215
            tunnel: w214 -> [w358]
            tunnel: [w357] -> w211
            tunnel: w210 -> [w357]
            tunnel: [w356] -> w199
            tunnel: w198 -> [w356]
            tunnel: [w355] -> w197
            tunnel: w196 -> [w355]
            tunnel: [w354] -> w195
            tunnel: w194 -> [w354]
            tunnel: [w353] -> w193
            tunnel: w192 -> [w353]
            tunnel: [w352] -> w152
            tunnel: w151 -> [w352]
            tunnel: [w351] -> w150
            tunnel: w149 -> [w351]
            tunnel: [w350] -> w130
            tunnel: w129 -> [w350]
            tunnel: [w393] -> w346
            tunnel: [w392] -> w344
            tunnel: [w388] -> w342
            tunnel: [w387] -> w337
            tunnel: [w386] -> w335
            tunnel: [w385] -> w302
            tunnel: [w384] -> w298
            tunnel: [w383] -> w278
            tunnel: [w382] -> w275
            tunnel: [w381] -> w273
            tunnel: [w380] -> w259
            tunnel: w257 -> [w393]
            tunnel: w256 -> [w392]
            tunnel: w255 -> [w391]
            tunnel: w254 -> [w387]
            tunnel: w253 -> [w386]
            tunnel: w252 -> [w383]
            tunnel: w251 -> [w382]
            tunnel: w250 -> [w381]
            tunnel: w249 -> [w385]
            tunnel: w248 -> [w384]
            tunnel: w247 -> [w380]
            tunnel: [w379] -> w230
            tunnel: w229 -> [w379]
            tunnel: w215 -> [w377]
            tunnel: [w377] -> w212
            tunnel: w211 -> [w378]
            tunnel: [w378] -> w208
            tunnel: w199 -> [w376]
            tunnel: w197 -> [w375]
            tunnel: w195 -> [w374]
            tunnel: w193 -> [w373]
            tunnel: [w376] -> w191
            tunnel: [w375] -> w187
            tunnel: [w374] -> w184
            tunnel: [w373] -> w183
            tunnel: w152 -> [w372]
            tunnel: w150 -> [w371]
            tunnel: [w372] -> w147
            tunnel: [w371] -> w145
            tunnel: w130 -> [_]
            tunnel: w346 -> [w1000]
            tunnel: [w1000] -> w345
            tunnel: w344 -> [w999]
            tunnel: [w999] -> w343
            tunnel: w342 -> [w995]
            tunnel: [w995] -> w341
            tunnel: w340 -> [w996]
            tunnel: [w996] -> w339
            tunnel: [w996] -> w338
            tunnel: w337 -> [w998]
            tunnel: [w998] -> w336
            tunnel: w335 -> [w997]
            tunnel: [w997] -> w334
            tunnel: [w996] -> w331
            tunnel: [w996] -> w317
            tunnel: w302 -> [w994]
            tunnel: [w994] -> w300
            tunnel: w298 -> [w993]
            tunnel: [w993] -> w295
            tunnel: [w992] -> w279
            tunnel: w278 -> [w992]
            tunnel: [w991] -> w276
            tunnel: w275 -> [w991]
            tunnel: [w990] -> w274
            tunnel: w273 -> [w990]
            tunnel: [w989] -> w260
            tunnel: w259 -> [w989]
            tunnel: [w988] -> w231
            tunnel: w230 -> [w988]
            tunnel: [w987] -> w213
            tunnel: w212 -> [w987]
            tunnel: [w986] -> w209
            tunnel: w208 -> [w986]
            tunnel: w191 -> [w985]
            tunnel: [w985] -> w190
            tunnel: [w984] -> w188
            tunnel: w187 -> [w984]
            tunnel: [w983] -> w186
            tunnel: w184 -> [w983]
            tunnel: w183 -> [w982]
            tunnel: [w982] -> w182
            tunnel: [w981] -> w148
            tunnel: w147 -> [w981]
            tunnel: [w980] -> w146
            tunnel: w145 -> [w980]
            tunnel: [w1023] -> w316
            tunnel: w345 -> [w1052]
            tunnel: w343 -> [w1051]
            tunnel: w341 -> [w1048]
            tunnel: w339 -> [w1047]
            tunnel: w338 -> [w1046]
            tunnel: w336 -> [w1036]
            tunnel: w334 -> [w1035]
            tunnel: w331 -> [w1037]
            tunnel: [w1033] -> w315
            tunnel: [w1034] -> w314
            tunnel: [w1045] -> w313
            tunnel: [w1044] -> w312
            tunnel: [w1043] -> w311
            tunnel: [w1042] -> w310
            tunnel: w317 -> [w1032]
            tunnel: [w1031] -> w309
            tunnel: [w1030] -> w308
            tunnel: [w1014] -> w307
            tunnel: [w1029] -> w306
            tunnel: w300 -> [w1028]
            tunnel: [w1028] -> w299
            tunnel: [w1027] -> w296
            tunnel: w295 -> [w1027]
            tunnel: w279 -> [w1026]
            tunnel: [w1026] -> w277
            tunnel: w276 -> [w1025]
            tunnel: w274 -> [w1024]
            tunnel: [w1025] -> w272
            tunnel: [w1024] -> w271
            tunnel: w260 -> [w1022]
            tunnel: [w1018] -> w232
            tunnel: w231 -> [w1018]
            tunnel: w213 -> [w1016]
            tunnel: w209 -> [w1015]
            tunnel: [w1009] -> w207
            tunnel: [w1014] -> w206
            tunnel: [w1012] -> w205
            tunnel: [w1010] -> w204
            tunnel: w190 -> [w1013]
            tunnel: [w1013] -> w189
            tunnel: w188 -> [w1012]
            tunnel: w186 -> [w1011]
            tunnel: [w1011] -> w185
            tunnel: w182 -> [w1010]
            tunnel: [w1009] -> w160
            tunnel: [w1008] -> w157
            tunnel: w148 -> [w1007]
            tunnel: w146 -> [w1006]
            tunnel: [w1003] -> w141
            tunnel: [w1001] -> w140
            tunnel: [w1003] -> w139
            tunnel: [w1002] -> w135
            tunnel: [w1001] -> w132
            tunnel: w316 -> [w1262]
            tunnel: [w1259] -> w290
            tunnel: w315 -> [w1275]
            tunnel: [w1275] -> w289
            tunnel: w314 -> [w1274]
            tunnel: [w1274] -> w288
            tunnel: w313 -> [w1273]
            tunnel: [w1273] -> w287
            tunnel: w312 -> [w1272]
            tunnel: [w1272] -> w286
            tunnel: w311 -> [w1271]
            tunnel: [w1271] -> w285
            tunnel: w310 -> [w1270]
            tunnel: [w1270] -> w284
            tunnel: [w1263] -> w283
            tunnel: w309 -> [w1256]
            tunnel: w308 -> [w1264]
            tunnel: w307 -> [w1263]
            tunnel: w306 -> [w1265]
            tunnel: [w1262] -> w282
            tunnel: w299 -> [w1261]
            tunnel: w296 -> [w1260]
            tunnel: [w1258] -> w281
            tunnel: [w1246] -> w280
            tunnel: w277 -> [w1257]
            tunnel: w272 -> [w1254]
            tunnel: w271 -> [w1253]
            tunnel: [w1255] -> w268
            tunnel: [w1252] -> w265
            tunnel: [w1251] -> w262
            tunnel: [w1247] -> w261
            tunnel: [w1245] -> w233
            tunnel: w232 -> [w1245]
            tunnel: w207 -> [w1244]
            tunnel: w206 -> [w1243]
            tunnel: w205 -> [w1242]
            tunnel: w204 -> [w1240]
            tunnel: [w1238] -> w203
            tunnel: [w1237] -> w202
            tunnel: [w1236] -> w201
            tunnel: [w1235] -> w200
            tunnel: w189 -> [w1239]
            tunnel: w185 -> [w1241]
            tunnel: [w1238] -> w181
            tunnel: [w1237] -> w180
            tunnel: [w1236] -> w179
            tunnel: [w1235] -> w178
            tunnel: [w1234] -> w161
            tunnel: w160 -> [w1234]
            tunnel: [w1233] -> w158
            tunnel: w157 -> [w1233]
            tunnel: w141 -> [w1232]
            tunnel: w140 -> [w1231]
            tunnel: w139 -> [w1230]
            tunnel: [w1230] -> w138
            tunnel: [w1229] -> w136
            tunnel: w135 -> [w1229]
            tunnel: w132 -> [w1228]
            tunnel: [w1228] -> w131
            tunnel: w290 -> [w1310]
            tunnel: [w1317] -> w330
            tunnel: [w1316] -> w329
            tunnel: w289 -> [w1316]
            tunnel: [w1311] -> w326
            tunnel: w288 -> [w1311]
            tunnel: [w1315] -> w324
            tunnel: w287 -> [w1315]
            tunnel: [w1314] -> w322
            tunnel: w286 -> [w1314]
            tunnel: [w1313] -> w320
            tunnel: w285 -> [w1313]
            tunnel: [w1312] -> w318
            tunnel: w284 -> [w1312]
            tunnel: w283 -> [w1299]
            tunnel: w282 -> [w1300]
            tunnel: w281 -> [w1297]
            tunnel: [w1297] -> w293
            tunnel: w280 -> [w1301]
            tunnel: [w1301] -> w291
            tunnel: [w1303] -> w269
            tunnel: w268 -> [w1303]
            tunnel: [w1304] -> w266
            tunnel: w265 -> [w1304]
            tunnel: [w1305] -> w263
            tunnel: w262 -> [w1305]
            tunnel: w261 -> [w1309]
            tunnel: [w1298] -> w234
            tunnel: w233 -> [w1298]
            tunnel: w203 -> [w1296]
            tunnel: w202 -> [w1295]
            tunnel: w201 -> [w1294]
            tunnel: w200 -> [w1293]
            tunnel: w181 -> [w1292]
            tunnel: w180 -> [w1291]
            tunnel: w179 -> [w1290]
            tunnel: w178 -> [w1289]
            tunnel: [w1292] -> w176
            tunnel: [w1291] -> w174
            tunnel: [w1290] -> w172
            tunnel: [w1289] -> w170
            tunnel: w161 -> [w1288]
            tunnel: [w1287] -> w159
            tunnel: w158 -> [w1287]
            tunnel: w138 -> [w1284]
            tunnel: [w1283] -> w137
            tunnel: w136 -> [w1283]
            tunnel: w131 -> [w1282]
            tunnel: w330 -> [w1334]
            tunnel: w329 -> [w1348]
            tunnel: w326 -> [w1342]
            tunnel: w324 -> [w1347]
            tunnel: w322 -> [w1344]
            tunnel: w320 -> [w1346]
            tunnel: w318 -> [w1345]
            tunnel: w293 -> [w1339]
            tunnel: w291 -> [w1338]
            tunnel: w269 -> [w1337]
            tunnel: w266 -> [w1336]
            tunnel: w263 -> [w1335]
            tunnel: [w1328] -> w154
            tunnel: [w1348] -> w246
            tunnel: [w1342] -> w245
            tunnel: [w1347] -> w244
            tunnel: [w1344] -> w243
            tunnel: [w1346] -> w242
            tunnel: [w1345] -> w241
            tunnel: [w1339] -> w240
            tunnel: [w1338] -> w239
            tunnel: [w1337] -> w238
            tunnel: [w1336] -> w237
            tunnel: [w1335] -> w236
            tunnel: [w1333] -> w235
            tunnel: w234 -> [w1333]
            tunnel: [w1332] -> w177
            tunnel: w176 -> [w1332]
            tunnel: [w1331] -> w175
            tunnel: w174 -> [w1331]
            tunnel: [w1330] -> w173
            tunnel: w172 -> [w1330]
            tunnel: [w1329] -> w171
            tunnel: w170 -> [w1329]
            tunnel: w159 -> [w1327]
            tunnel: [w1326] -> w144
            tunnel: [w1325] -> w143
            tunnel: w137 -> [w1324]
            tunnel: [w1323] -> w134
            tunnel: [w1322] -> w133
            tunnel: w246 -> [w1396]
            tunnel: w245 -> [w1395]
            tunnel: w244 -> [w1394]
            tunnel: w243 -> [w1393]
            tunnel: w242 -> [w1392]
            tunnel: w241 -> [w1391]
            tunnel: w240 -> [w1390]
            tunnel: w239 -> [w1389]
            tunnel: w238 -> [w1388]
            tunnel: w237 -> [w1387]
            tunnel: w236 -> [w1386]
            tunnel: w235 -> [w1380]
            tunnel: [w1396] -> w228
            tunnel: [w1395] -> w227
            tunnel: [w1394] -> w226
            tunnel: [w1393] -> w225
            tunnel: [w1392] -> w224
            tunnel: [w1391] -> w223
            tunnel: [w1390] -> w222
            tunnel: [w1389] -> w221
            tunnel: [w1388] -> w220
            tunnel: [w1387] -> w219
            tunnel: [w1386] -> w218
            tunnel: [w1380] -> w217
            tunnel: [w1379] -> w216
            tunnel: w177 -> [w1377]
            tunnel: w175 -> [w1376]
            tunnel: w173 -> [w1375]
            tunnel: w171 -> [w1374]
            tunnel: [w1377] -> w169
            tunnel: [w1376] -> w167
            tunnel: [w1375] -> w165
            tunnel: [w1374] -> w163
            tunnel: w144 -> [w1373]
            tunnel: w143 -> [w1372]
            tunnel: [w1367] -> w142
            tunnel: w134 -> [w1366]
            tunnel: w133 -> [w1365]
            tunnel: [w1407] -> w264
            tunnel: [w1408] -> w267
            tunnel: [w1409] -> w270
            tunnel: [w1410] -> w292
            tunnel: [w1411] -> w294
            tunnel: [w1412] -> w319
            tunnel: [w1413] -> w321
            tunnel: [w1414] -> w323
            tunnel: [w1415] -> w325
            tunnel: [w1416] -> w327
            tunnel: [w1417] -> w328
            tunnel: w228 -> [w1417]
            tunnel: w227 -> [w1416]
            tunnel: w226 -> [w1415]
            tunnel: w225 -> [w1414]
            tunnel: w224 -> [w1413]
            tunnel: w223 -> [w1412]
            tunnel: w222 -> [w1411]
            tunnel: w221 -> [w1410]
            tunnel: w220 -> [w1409]
            tunnel: w219 -> [w1408]
            tunnel: w218 -> [w1407]
            tunnel: w217 -> [w1403]
            tunnel: w216 -> [w1402]
            tunnel: [w1401] -> w168
            tunnel: w169 -> [w1401]
            tunnel: [w1400] -> w166
            tunnel: w167 -> [w1400]
            tunnel: [w1399] -> w164
            tunnel: w165 -> [w1399]
            tunnel: [w1398] -> w162
            tunnel: w163 -> [w1398]
            tunnel: [w1397] -> w156
            tunnel: w142 -> [w1397]
            frame #0 {
              n19 = Tick Count (ms)() -> (millisecond timer value=w359:u32)
            }
            frame #1 {
              n20 = while {
                tunnel: w391 -> [w398]
                tunnel: [w397] -> w390
                tunnel: [w396] -> w389
                tunnel: w377 -> [w394]
                stop <- w399 stop-if-true
                n21 = event shown="[12] \"Ramp\": Value Change" {
                  selector: _ -> [_ _ _ _ _ _ _ _ _ _ _ _ _ _]
                  dyn-events: _ -> [_ _ _ _ _ _ _ _ _ _ _ _ _ _]
                  timeout: 1 -> [_ _ _ _ _ _ _ _ _ _ _ _ _ _]
                  tunnel: [TRUE ("Set Gauge to Zero") w407 w456 w477 w503 w538 w594 w645 w724 w795 "Set Gauge to Zero" _ _ "Get SetPoint"] -> w399
                  tunnel: w398 -> [w403 w406 w453 w475 w499 w537 w590 w643 w722 w793 w870 w892 w900 w972]
                  tunnel: [w402 w405 w452 w474 w501 w535 w592 w642 w721 w792 w869 w891 w899 w971] -> w397
                  tunnel: [w401 w404 w451 w473 w500 w536 w591 w641 w720 w791 w868 w890 w898 w970] -> w396
                  tunnel: w394 -> [_ _ _ _ _ _ _ _ _ _ w866 _ _ _]
                  event Timeout {
                    n22 = event-data() -> ()  [unwired: 1 in, 1 out]
                    n23 = Unbundle(w403) -> ("VISA resource name out"=w402:refnum<visa-resource-name>, "error out"=w401:errorcluster)  [unwired: 2 out]
                  }
                  event "Setpoint\n START": Value Change {
                    n24 = event-data() -> ()  [unwired: 1 in, 1 out]
                    n25 = stacked-sequence {
                      tunnel: w406 -> [_ w413 _]
                      tunnel: [_ w412 _] -> w404
                      tunnel: [_ w411 _] -> w405
                      frame #0 {
                        n26 = property on="Setpoint\n START" class="Bool"("Blinking"=TRUE) -> ()  [unwired: 2 in, 2 out]
                        n27 = property on="ON" class="Bool (strict)"("Blinking"=FALSE) -> ()  [unwired: 2 in, 2 out]
                      }
                      frame #1 {
                        n28 = for {
                          N: 2 -> [_]
                          tunnel: w413 -> [w417]
                          tunnel: [w416] -> w412
                          tunnel: [w415] -> w411
                          i -> [w419]
                          n29 = flat-sequence {
                            tunnel: [w422] -> w418
                            tunnel: w419 -> [w421]
                            tunnel: [w440] -> w420
                            tunnel: w418 -> [w439]
                            tunnel: w417 -> [w441]
                            tunnel: [w438] -> w416
                            tunnel: [w437] -> w415
                            tunnel: w420 -> [w447]
                            tunnel: w419 -> [w446]
                            frame #0 {
                              n30 = case shown="0, Default" w421 {
                                tunnel: [w431 w433] -> w422
                                frame 0, Default {
                                n31 = Multiply(x=10.0, y="SP 1 input (°C)") -> (x*y=w428:dbl)
                                n32 = local read "RAM"() -> (w426:bool)
                                n33 = Number To Hexadecimal String(1:i16 5 ("width (-)"), 2:w428) -> (0:w430:string)
                                n34 = Select(t="*P012", s=w426, f="*P012") -> (s? t:f=w423:string)
                                n35 = Concatenate Strings(w423, w430) -> (w431:string)
                                }
                                frame 1 {
                                n36 = local read "RAM"() -> (w436:bool)
                                n37 = Select(t="*G01", s=w436, f="*R01") -> (s? t:f=w433:string)
                                }
                              }
                            }
                            frame #1 {
                              n38 = Unbundle(w441) -> ("VISA resource name out"=w442:refnum<visa-resource-name>, "error out"=w444:errorcluster, "Delay (ms)"=w443:u32, "Write/\nRead"=w445:bool)
                              n39 = call "I3252_Comm_Interface.vi"("VISA resource name in"=w442, "error in"=w444, "Delay (ms)"=w443, "Write"=w445, "String to Write"=w439, "Read"=w445) -> ("VISA resource name out"=w437:refnum<visa-resource-name>, "error out"=w438:errorcluster, "Read String"=w440:string)  [unwired: 2 in]
                            }
                            frame #2 {
                              n40 = case shown="0, Default" w446 {
                                tunnel: w447 -> [_ w449]
                                frame 0, Default {
                                }
                                frame 1 {
                                n41 = call "I3252_Edit_Setpoint.vi"("Read String"=w449) -> ("Setpoint is"=→"SP 1 is (°C)":dbl)
                                }
                              }
                            }
                          }
                        }
                      }
                      frame #2 {
                        n42 = property on="Setpoint\n START" class="Bool"("Blinking"=FALSE) -> ()  [unwired: 2 in, 2 out]
                      }
                    }
                    n43 = Not(x="Setpoint\n START") -> (.not. x?=w407:bool)
                  }
                  event "Standby": Value Change {
                    n44 = event-data() -> ()  [unwired: 1 in, 1 out]
                    n45 = flat-sequence {
                      tunnel: [w464] -> w454
                      tunnel: w454 -> [w468]
                      tunnel: w453 -> [w467]
                      tunnel: [w466] -> w451
                      tunnel: [w465] -> w452
                      frame #0 {
                        n46 = local read "Standby"() -> (w457:bool)
                        n47 = Select(t=TRUE, s=w457, f=FALSE) -> (s? t:f=w460:bool)
                        n48 = property on="Standby" class="Bool (strict)"("Blinking"=w460) -> ()  [unwired: 2 in, 2 out]
                      }
                      frame #1 {
                        n49 = local read "Standby"() -> (w462:bool)
                        n50 = Select(t="*D03", s=w462, f="*E03") -> (s? t:f=w464:string)
                      }
                      frame #2 {
                        n51 = Unbundle(w467) -> ("VISA resource name out"=w469:refnum<visa-resource-name>, "error out"=w471:errorcluster, "Delay (ms)"=w470:u32, "Write/\nRead"=w472:bool)
                        n52 = call "I3252_Comm_Interface.vi"("VISA resource name in"=w469, "error in"=w471, "Delay (ms)"=w470, "Write"=w472, "String to Write"=w468, "Read"=w472) -> ("VISA resource name out"=w465:refnum<visa-resource-name>, "error out"=w466:errorcluster)  [unwired: 2 in, 1 out]
                      }
                    }
                    n53 = Not(x="Standby") -> (.not. x?=w456:bool)
                  }
                  event "Set Command": Value Change {
                    n54 = event-data() -> ()  [unwired: 1 in, 1 out]
                    n55 = stacked-sequence {
                      tunnel: w475 -> [_ w482 _]
                      tunnel: [_ w481 _] -> w474
                      tunnel: [_ w480 _] -> w473
                      frame #0 {
                        n56 = property on="Set Command" class="Bool"("Blinking"=TRUE) -> ()  [unwired: 2 in, 2 out]
                        n57 = property on="ON" class="Bool (strict)"("Blinking"=FALSE) -> ()  [unwired: 2 in, 2 out]
                      }
                      frame #1 {
                        n58 = flat-sequence {
                          tunnel: [w487] -> w484
                          tunnel: [w490] -> w483
                          tunnel: w484 -> [w491]
                          tunnel: w482 -> [w492]
                          tunnel: [w489] -> w481
                          tunnel: [w488] -> _
                          tunnel: [w488] -> w480
                          tunnel: w483 -> [w497]
                          frame #0 {
                            n59 = Concatenate Strings("*", "Command input") -> (w487:string)
                          }
                          frame #1 {
                            n60 = Unbundle(w492) -> ("VISA resource name out"=w496:refnum<visa-resource-name>, "error out"=w494:errorcluster, "Delay (ms)"=w495:u32, "Write/\nRead"=w493:bool)
                            n61 = call "I3252_Comm_Interface.vi"("VISA resource name in"=w496, "error in"=w494, "Delay (ms)"=w495, "Write"=w493, "String to Write"=w491, "Read"=w493) -> ("VISA resource name out"=w489:refnum<visa-resource-name>, "error out"=w488:errorcluster, "Read String"=w490:string)  [unwired: 2 in]
                          }
                          frame #2 {
                            "Command output" <- w497
                          }
                        }
                      }
                      frame #2 {
                        n62 = property on="Set Command" class="Bool"("Blinking"=FALSE) -> ()  [unwired: 2 in, 2 out]
                      }
                    }
                    n63 = Not(x="Set Command") -> (.not. x?=w477:bool)
                  }
                  event "Reset\nSTOPP": Value Change {
                    n64 = event-data() -> ()  [unwired: 1 in, 1 out]
                    n65 = stacked-sequence {
                      tunnel: [_ w510 _] -> w500
                      tunnel: [_ w509 _] -> w501
                      tunnel: w499 -> [_ w507 _]
                      frame #0 {
                        n66 = property on="Reset\nSTOPP" class="Bool"("Blinking"=FALSE) -> ()  [unwired: 2 in, 2 out]
                        n67 = property on="ON" class="Bool (strict)"("Blinking"=FALSE) -> ()  [unwired: 2 in, 2 out]
                      }
                      frame #1 {
                        n68 = for {
                          N: 2 -> [_]
                          tunnel: [w516] -> w510
                          tunnel: [w515] -> w509
                          tunnel: w507 -> [w514]
                          i -> [w512]
                          n69 = flat-sequence {
                            tunnel: w512 -> [w518]
                            tunnel: [w517] -> w513
                            tunnel: [w523] -> w516
                            tunnel: [w524] -> w515
                            tunnel: w514 -> [w525]
                            tunnel: w513 -> [w522]
                            tunnel: [w521] -> w511
                            tunnel: w512 -> [w531]
                            tunnel: w511 -> [w530]
                            frame #0 {
                              n70 = case shown="0, Default" w518 {
                                tunnel: ["*Z02" "*G01"] -> w517
                                frame 0, Default {
                                }
                                frame 1 {
                                }
                              }
                            }
                            frame #1 {
                              n71 = Unbundle(w525) -> ("VISA resource name out"=w526:refnum<visa-resource-name>, "error out"=w528:errorcluster, "Delay (ms)"=w527:u32, "Write/\nRead"=w529:bool)
                              n72 = call "I3252_Comm_Interface.vi"("VISA resource name in"=w526, "error in"=w528, "Delay (ms)"=w527, "Write"=w529, "String to Write"=w522, "Read"=w529) -> ("VISA resource name out"=w524:refnum<visa-resource-name>, "error out"=w523:errorcluster, "Read String"=w521:string)  [unwired: 2 in]
                            }
                            frame #2 {
                              n73 = case shown="0, Default" w531 {
                                tunnel: w530 -> [_ w533]
                                frame 0, Default {
                                }
                                frame 1 {
                                n74 = call "I3252_Edit_Setpoint.vi"("Read String"=w533) -> ("Setpoint is"=w532:dbl)
                                n75 = local write "SP 1 is (°C)"(w532) -> ()
                                }
                              }
                            }
                          }
                        }
                        n76 = Wait (ms)(milliseconds to wait=u32 4000) -> ()  [unwired: 1 out]
                      }
                      frame #2 {
                        n77 = property on="Reset\nSTOPP" class="Bool"("Blinking"=FALSE) -> ()  [unwired: 2 in, 2 out]
                      }
                    }
                    n78 = Not(x="Reset\nSTOPP") -> (.not. x?=w503:bool)
                  }
                  event "Auto Tune": Value Change {
                    n79 = event-data() -> ()  [unwired: 1 in, 1 out]
                    n80 = stacked-sequence {
                      tunnel: w537 -> [_ w544 w589]
                      tunnel: [_ w543 _] -> w536
                      tunnel: [_ w542 _] -> w535
                      frame #0 {
                        n81 = property on="Auto Tune" class="Bool"("Blinking"=TRUE) -> ()  [unwired: 2 in, 2 out]
                        n82 = property on="ON" class="Bool (strict)"("Blinking"=FALSE) -> ()  [unwired: 2 in, 2 out]
                      }
                      frame #1 {
                        n83 = for {
                          N: 4 -> [_]
                          tunnel: [w549] -> w542
                          tunnel: [w548] -> w543
                          tunnel: w544 -> [w547]
                          i -> [w552]
                          n84 = flat-sequence {
                            tunnel: w552 -> [w554]
                            tunnel: [w553] -> w550
                            tunnel: w550 -> [w569]
                            tunnel: [w568] -> w551
                            tunnel: [w571] -> w549
                            tunnel: [w570] -> w548
                            tunnel: w547 -> [w567]
                            tunnel: w552 -> [w577]
                            tunnel: w551 -> [w576]
                            frame #0 {
                              n85 = case shown="0, Default" w554 {
                                tunnel: ["*V01" w557 "*W0C35" "*Z02"] -> w553
                                frame 0, Default {
                                }
                                frame 1 {
                                n86 = local read "(°C)"() -> (w556:dbl)
                                n87 = Add(x=20.0, y=w556) -> (x+y=w563:dbl)
                                n88 = Multiply(x=10.0, y=w563) -> (x*y=w560:dbl)
                                n89 = Number To Hexadecimal String(1:i16 5 ("width (-)"), 2:w560) -> (0:w559:string)
                                n90 = Concatenate Strings("*W012", w559) -> (w557:string)
                                }
                                frame 2 {
                                # "35 hex = \n00110101 bin"
                                }
                                frame 3 {
                                }
                              }
                            }
                            frame #1 {
                              n91 = Unbundle(w567) -> ("VISA resource name out"=w575:refnum<visa-resource-name>, "error out"=w573:errorcluster, "Delay (ms)"=w574:u32, "Write/\nRead"=w572:bool)
                              n92 = call "I3252_Comm_Interface.vi"("VISA resource name in"=w575, "error in"=w573, "Delay (ms)"=w574, "Write"=w572, "String to Write"=w569, "Read"=w572) -> ("VISA resource name out"=w571:refnum<visa-resource-name>, "error out"=w570:errorcluster, "Read String"=w568:string)  [unwired: 2 in]
                            }
                            frame #2 {
                              n93 = case shown="0, Default" w577 {
                                tunnel: w576 -> [w579]
                                frame 0, Default {
                                n94 = call <vilib>:"Space Constant.vi"() -> ("String"=w582:string)
                                n95 = Search/Split String(string=w579, search string/char (-)=w582) -> (match + rest of string=w581:string)  [unwired: 1 in, 2 out]
                                n96 = Fract/Exp String To Number(use system decimal point (T)=FALSE, string=w581) -> (number=w578:dbl)  [unwired: 2 in, 1 out]
                                n97 = local write "(°C)"(w578) -> ()
                                }
                              }
                            }
                          }
                        }
                        n98 = Wait (ms)(milliseconds to wait=u32 45000) -> ()  [unwired: 1 out]
                      }
                      frame #2 {
                        n99 = Unbundle(w589) -> ("VISA resource name out"=w588:refnum<visa-resource-name>, "error out"=w586:errorcluster, "Delay (ms)"=w587:u32, "Write/\nRead"=w585:bool)
                        n100 = property on="Auto Tune" class="Bool"("Blinking"=FALSE) -> ()  [unwired: 2 in, 2 out]
                        n101 = call "I3252_Comm_Interface.vi"("VISA resource name in"=w588, "error in"=w586, "Delay (ms)"=w587, "Write"=w585, "String to Write"="*W01200000", "Read"=w585) -> ()  [unwired: 2 in, 3 out]
                      }
                    }
                    n102 = Not(x="Auto Tune") -> (.not. x?=w538:bool)
                  }
                  event "Write LOW/HI": Value Change {
                    n103 = event-data() -> ()  [unwired: 1 in, 1 out]
                    n104 = stacked-sequence {
                      tunnel: [_ w599 _] -> w592
                      tunnel: [_ w598 _] -> w591
                      tunnel: w590 -> [_ w597 _]
                      frame #0 {
                        n105 = property on="Write LOW/HI" class="Bool"("Blinking"=TRUE) -> ()  [unwired: 2 in, 2 out]
                        n106 = property on="ON" class="Bool (strict)"("Blinking"=FALSE) -> ()  [unwired: 2 in, 2 out]
                      }
                      frame #1 {
                        n107 = for {
                          N: 4 -> [_]
                          tunnel: [w603] -> w599
                          tunnel: [w602] -> w598
                          tunnel: w597 -> [w601]
                          i -> [w605]
                          n108 = flat-sequence {
                            tunnel: w605 -> [w607]
                            tunnel: [w608] -> w604
                            tunnel: w604 -> [w622]
                            tunnel: [w623] -> w606
                            tunnel: [w625] -> w603
                            tunnel: [w624] -> w602
                            tunnel: w601 -> [w621]
                            tunnel: w606 -> [w631]
                            tunnel: w605 -> [w630]
                            frame #0 {
                              n109 = case shown="1" w607 {
                                tunnel: [w610 w616 "*R27" "*R28"] -> w608
                                frame 0, Default {
                                n110 = Number To Hexadecimal String(1:i16 2 ("width (-)"), 2:"% LOW Sollwert") -> (0:w611:string)
                                n111 = Concatenate Strings("*W27", w611) -> (w610:string)
                                }
                                frame 1 {
                                n112 = Number To Hexadecimal String(1:i16 2 ("width (-)"), 2:"% High Sollwert") -> (0:w617:string)
                                n113 = Concatenate Strings("*W28", w617) -> (w616:string)
                                }
                                frame 2 {
                                }
                                frame 3 {
                                }
                              }
                            }
                            frame #1 {
                              n114 = Unbundle(w621) -> ("VISA resource name out"=w629:refnum<visa-resource-name>, "error out"=w627:errorcluster, "Delay (ms)"=w628:u32, "Write/\nRead"=w626:bool)
                              n115 = call "I3252_Comm_Interface.vi"("VISA resource name in"=w629, "error in"=w627, "Delay (ms)"=w628, "Write"=w626, "String to Write"=w622, "Read"=w626) -> ("VISA resource name out"=w625:refnum<visa-resource-name>, "error out"=w624:errorcluster, "Read String"=w623:string)  [unwired: 2 in]
                            }
                            frame #2 {
                              n116 = case shown="0, Default" w630 {
                                tunnel: w631 -> [_ w635 w639]
                                frame 0, Default {
                                }
                                frame 2 {
                                n117 = String Subset(string=w635, offset (0)=3) -> (substring=w633:string)  [unwired: 1 in]
                                n118 = Hexadecimal String To Number(string=w633) -> (number=→"% LOW Istwert":u32)  [unwired: 2 in, 1 out]
                                }
                                frame 3 {
                                n119 = String Subset(string=w639, offset (0)=3) -> (substring=w637:string)  [unwired: 1 in]
                                n120 = Hexadecimal String To Number(string=w637) -> (number=→"% HIGH Istwert":u32)  [unwired: 2 in, 1 out]
                                }
                              }
                            }
                          }
                        }
                      }
                      frame #2 {
                        n121 = property on="Write LOW/HI" class="Bool"("Blinking"=FALSE) -> ()  [unwired: 2 in, 2 out]
                      }
                    }
                    n122 = Not(x="Write LOW/HI") -> (.not. x?=w594:bool)
                  }
                  event "Set PID": Value Change {
                    n123 = event-data() -> ()  [unwired: 1 in, 1 out]
                    n124 = stacked-sequence {
                      tunnel: w643 -> [_ w650 _]
                      tunnel: [_ w649 _] -> w642
                      tunnel: [_ w648 _] -> w641
                      frame #0 {
                        n125 = property on="Set PID" class="Bool"("Blinking"=TRUE) -> ()  [unwired: 2 in, 2 out]
                        n126 = property on="ON" class="Bool (strict)"("Blinking"=FALSE) -> ()  [unwired: 2 in, 2 out]
                      }
                      frame #1 {
                        n127 = for {
                          N: 6 -> [_]
                          tunnel: w650 -> [w654]
                          tunnel: [w653] -> w649
                          tunnel: [w652] -> w648
                          i -> [w656]
                          n128 = flat-sequence {
                            tunnel: w656 -> [w658]
                            tunnel: [w659] -> w655
                            tunnel: w655 -> [w700]
                            tunnel: [w696] -> w657
                            tunnel: w654 -> [w699]
                            tunnel: [w698] -> w652
                            tunnel: [w697] -> w653
                            tunnel: w657 -> [w706]
                            tunnel: w656 -> [w705]
                            frame #0 {
                              n129 = case shown="0, Default" w658 {
                                tunnel: [w666 w674 w682 w684 w688 w692] -> w659
                                frame 0, Default {
                                n130 = local read "RAM"() -> (w660:bool)
                                n131 = Number To Hexadecimal String(1:i16 4 ("width (-)"), 2:"P (PB1) Sollwert") -> (0:w667:string)
                                n132 = Select(t="*P17", s=w660, f="*W17") -> (s? t:f=w661:string)
                                n133 = Concatenate Strings(w661, w667) -> (w666:string)
                                }
                                frame 1 {
                                n134 = local read "RAM"() -> (w668:bool)
                                n135 = Number To Hexadecimal String(1:i16 4 ("width (-)"), 2:"I ( Reset1) Sollwert") -> (0:w675:string)
                                n136 = Select(t="*P18", s=w668, f="*W18") -> (s? t:f=w670:string)
                                n137 = Concatenate Strings(w670, w675) -> (w674:string)
                                }
                                frame 2 {
                                n138 = local read "RAM"() -> (w677:bool)
                                n139 = Number To Hexadecimal String(1:i16 4 ("width (-)"), 2:"D (Rate) Sollwert") -> (0:w683:string)
                                n140 = Select(t="*P19", s=w677, f="*W19") -> (s? t:f=w678:string)
                                n141 = Concatenate Strings(w678, w683) -> (w682:string)
                                }
                                frame 3 {
                                n142 = local read "RAM"() -> (w687:bool)
                                n143 = Select(t="*G17", s=w687, f="*R17") -> (s? t:f=w684:string)
                                }
                                frame 4 {
                                n144 = local read "RAM"() -> (w691:bool)
                                n145 = Select(t="*G18", s=w691, f="*R18") -> (s? t:f=w688:string)
                                }
                                frame 5 {
                                n146 = local read "RAM"() -> (w695:bool)
                                n147 = Select(t="*G19", s=w695, f="*R19") -> (s? t:f=w692:string)
                                }
                              }
                            }
                            frame #1 {
                              n148 = Unbundle(w699) -> ("VISA resource name out"=w704:refnum<visa-resource-name>, "error out"=w702:errorcluster, "Delay (ms)"=w703:u32, "Write/\nRead"=w701:bool)
                              n149 = call "I3252_Comm_Interface.vi"("VISA resource name in"=w704, "error in"=w702, "Delay (ms)"=w703, "Write"=w701, "String to Write"=w700, "Read"=w701) -> ("VISA resource name out"=w697:refnum<visa-resource-name>, "error out"=w698:errorcluster, "Read String"=w696:string)  [unwired: 2 in]
                            }
                            frame #2 {
                              n150 = case shown="5" w705 {
                                tunnel: w706 -> [_ w710 w714 w718]
                                frame 0, Default {
                                }
                                frame 3 {
                                n151 = String Subset(string=w710, offset (0)=3) -> (substring=w708:string)  [unwired: 1 in]
                                n152 = Hexadecimal String To Number(string=w708) -> (number=→"P (PB1) Istwert":u32)  [unwired: 2 in, 1 out]
                                }
                                frame 4 {
                                n153 = String Subset(string=w714, offset (0)=3) -> (substring=w712:string)  [unwired: 1 in]
                                n154 = Hexadecimal String To Number(string=w712) -> (number=→"I ( Reset1) Istwert":u32)  [unwired: 2 in, 1 out]
                                }
                                frame 5 {
                                n155 = String Subset(string=w718, offset (0)=3) -> (substring=w716:string)  [unwired: 1 in]
                                n156 = Hexadecimal String To Number(string=w716) -> (number=→"D (Rate) IstWert":u32)  [unwired: 2 in, 1 out]
                                }
                              }
                            }
                          }
                        }
                      }
                      frame #2 {
                        n157 = property on="Set PID" class="Bool"("Blinking"=FALSE) -> ()  [unwired: 2 in, 2 out]
                      }
                    }
                    n158 = Not(x="Set PID") -> (.not. x?=w645:bool)
                  }
                  event "Get Values": Value Change {
                    n159 = event-data() -> ()  [unwired: 1 in, 1 out]
                    n160 = stacked-sequence {
                      tunnel: w722 -> [_ w729 _]
                      tunnel: [_ w728 _] -> w721
                      tunnel: [_ w727 _] -> w720
                      frame #0 {
                        n161 = property on="Get Values" class="Bool"("Blinking"=TRUE) -> ()  [unwired: 2 in, 2 out]
                        n162 = property on="ON" class="Bool (strict)"("Blinking"=FALSE) -> ()  [unwired: 2 in, 2 out]
                      }
                      frame #1 {
                        n163 = for {
                          N: 6 -> [_]
                          tunnel: w729 -> [w733]
                          tunnel: [w732] -> w728
                          tunnel: [w731] -> w727
                          i -> [w735]
                          n164 = flat-sequence {
                            tunnel: w735 -> [w737]
                            tunnel: [w738] -> w734
                            tunnel: w734 -> [w760]
                            tunnel: [w761] -> w736
                            tunnel: w733 -> [w759]
                            tunnel: [w758] -> w731
                            tunnel: [w757] -> w732
                            tunnel: w736 -> [w767]
                            tunnel: w735 -> [w766]
                            frame #0 {
                              n165 = case shown="0, Default" w737 {
                                tunnel: [w741 w745 w749 "*R27" "*R28" w755] -> w738
                                frame 0, Default {
                                n166 = local read "RAM"() -> (w742:bool)
                                n167 = Select(t="*G17", s=w742, f="*R17") -> (s? t:f=w741:string)
                                }
                                frame 1 {
                                n168 = local read "RAM"() -> (w746:bool)
                                n169 = Select(t="*G18", s=w746, f="*R18") -> (s? t:f=w745:string)
                                }
                                frame 2 {
                                n170 = local read "RAM"() -> (w750:bool)
                                n171 = Select(t="*G19", s=w750, f="*R19") -> (s? t:f=w749:string)
                                }
                                frame 3 {
                                }
                                frame 4 {
                                }
                                frame 5 {
                                n172 = local read "RAM"() -> (w756:bool)
                                n173 = Select(t="*G01", s=w756, f="*R01") -> (s? t:f=w755:string)
                                }
                              }
                            }
                            frame #1 {
                              n174 = Unbundle(w759) -> ("VISA resource name out"=w765:refnum<visa-resource-name>, "error out"=w763:errorcluster, "Delay (ms)"=w764:u32, "Write/\nRead"=w762:bool)
                              n175 = call "I3252_Comm_Interface.vi"("VISA resource name in"=w765, "error in"=w763, "Delay (ms)"=w764, "Write"=w762, "String to Write"=w760, "Read"=w762) -> ("VISA resource name out"=w757:refnum<visa-resource-name>, "error out"=w758:errorcluster, "Read String"=w761:string)  [unwired: 2 in]
                            }
                            frame #2 {
                              n176 = case shown="0, Default" w766 {
                                tunnel: w767 -> [w769 w773 w777 w781 w785 w789]
                                frame 0, Default {
                                n177 = String Subset(string=w769, offset (0)=3) -> (substring=w770:string)  [unwired: 1 in]
                                n178 = Hexadecimal String To Number(string=w770) -> (number=w768:u32)  [unwired: 2 in, 1 out]
                                n179 = local write "P (PB1) Sollwert"(w768) -> ()
                                n180 = local write "P (PB1) Istwert"(w768) -> ()
                                }
                                frame 1 {
                                n181 = String Subset(string=w773, offset (0)=3) -> (substring=w774:string)  [unwired: 1 in]
                                n182 = Hexadecimal String To Number(string=w774) -> (number=w772:u32)  [unwired: 2 in, 1 out]
                                n183 = local write "I ( Reset1) Sollwert"(w772) -> ()
                                n184 = local write "I ( Reset1) Istwert"(w772) -> ()
                                }
                                frame 2 {
                                n185 = String Subset(string=w777, offset (0)=3) -> (substring=w778:string)  [unwired: 1 in]
                                n186 = Hexadecimal String To Number(string=w778) -> (number=w776:u32)  [unwired: 2 in, 1 out]
                                n187 = local write "D (Rate) Sollwert"(w776) -> ()
                                n188 = local write "D (Rate) IstWert"(w776) -> ()
                                }
                                frame 3 {
                                n189 = String Subset(string=w781, offset (0)=3) -> (substring=w782:string)  [unwired: 1 in]
                                n190 = Hexadecimal String To Number(string=w782) -> (number=w780:u32)  [unwired: 2 in, 1 out]
                                n191 = local write "% LOW Istwert"(w780) -> ()
                                n192 = local write "% LOW Sollwert"(w780) -> ()
                                }
                                frame 4 {
                                n193 = String Subset(string=w785, offset (0)=3) -> (substring=w786:string)  [unwired: 1 in]
                                n194 = Hexadecimal String To Number(string=w786) -> (number=w784:u32)  [unwired: 2 in, 1 out]
                                n195 = local write "% High Sollwert"(w784) -> ()
                                n196 = local write "% HIGH Istwert"(w784) -> ()
                                }
                                frame 5 {
                                n197 = call "I3252_Edit_Setpoint.vi"("Read String"=w789) -> ("Setpoint is"=w788:dbl)
                                n198 = local write "SP 1 is (°C)"(w788) -> ()
                                }
                              }
                            }
                          }
                        }
                      }
                      frame #2 {
                        n199 = property on="Get Values" class="Bool"("Blinking"=FALSE) -> ()  [unwired: 2 in, 2 out]
                      }
                    }
                    n200 = Not(x="Get Values") -> (.not. x?=w724:bool)
                  }
                  event "RAM": Value Change {
                    n201 = event-data() -> ()  [unwired: 1 in, 1 out]
                    n202 = stacked-sequence {
                      tunnel: w793 -> [_ w800 _]
                      tunnel: [_ w799 _] -> w792
                      tunnel: [_ w798 _] -> w791
                      frame #0 {
                        n203 = property on="RAM" class="Bool (strict)"("Blinking"=TRUE) -> ()  [unwired: 2 in, 2 out]
                        n204 = property on="ON" class="Bool (strict)"("Blinking"=FALSE) -> ()  [unwired: 2 in, 2 out]
                      }
                      frame #1 {
                        n205 = for {
                          N: 6 -> [_]
                          tunnel: w800 -> [w804]
                          tunnel: [w803] -> w799
                          tunnel: [w802] -> w798
                          i -> [w806]
                          n206 = flat-sequence {
                            tunnel: w806 -> [w808]
                            tunnel: [w809] -> w805
                            tunnel: w805 -> [w828]
                            tunnel: [w829] -> w807
                            tunnel: w804 -> [w832]
                            tunnel: [w831] -> w802
                            tunnel: [w830] -> w803
                            tunnel: w807 -> [w838]
                            tunnel: w806 -> [w837]
                            frame #0 {
                              n207 = case shown="0, Default" w808 {
                                tunnel: [w812 w816 w820 "*R27" "*R28" w826] -> w809
                                frame 0, Default {
                                n208 = local read "RAM"() -> (w813:bool)
                                n209 = Select(t="*G17", s=w813, f="*R17") -> (s? t:f=w812:string)
                                }
                                frame 1 {
                                n210 = local read "RAM"() -> (w817:bool)
                                n211 = Select(t="*G18", s=w817, f="*R18") -> (s? t:f=w816:string)
                                }
                                frame 2 {
                                n212 = local read "RAM"() -> (w821:bool)
                                n213 = Select(t="*G19", s=w821, f="*R19") -> (s? t:f=w820:string)
                                }
                                frame 3 {
                                }
                                frame 4 {
                                }
                                frame 5 {
                                n214 = local read "RAM"() -> (w827:bool)
                                n215 = Select(t="*G01", s=w827, f="*R01") -> (s? t:f=w826:string)
                                }
                              }
                            }
                            frame #1 {
                              n216 = Unbundle(w832) -> ("VISA resource name out"=w836:refnum<visa-resource-name>, "error out"=w834:errorcluster, "Delay (ms)"=w835:u32, "Write/\nRead"=w833:bool)
                              n217 = call "I3252_Comm_Interface.vi"("VISA resource name in"=w836, "error in"=w834, "Delay (ms)"=w835, "Write"=w833, "String to Write"=w828, "Read"=w833) -> ("VISA resource name out"=w830:refnum<visa-resource-name>, "error out"=w831:errorcluster, "Read String"=w829:string)  [unwired: 2 in]
                            }
                            frame #2 {
                              n218 = case shown="0, Default" w837 {
                                tunnel: w838 -> [w840 w844 w848 w852 w856 w860]
                                frame 0, Default {
                                n219 = String Subset(string=w840, offset (0)=3) -> (substring=w841:string)  [unwired: 1 in]
                                n220 = Hexadecimal String To Number(string=w841) -> (number=w839:u32)  [unwired: 2 in, 1 out]
                                n221 = local write "P (PB1) Sollwert"(w839) -> ()
                                n222 = local write "P (PB1) Istwert"(w839) -> ()
                                }
                                frame 1 {
                                n223 = String Subset(string=w844, offset (0)=3) -> (substring=w845:string)  [unwired: 1 in]
                                n224 = Hexadecimal String To Number(string=w845) -> (number=w843:u32)  [unwired: 2 in, 1 out]
                                n225 = local write "I ( Reset1) Sollwert"(w843) -> ()
                                n226 = local write "I ( Reset1) Istwert"(w843) -> ()
                                }
                                frame 2 {
                                n227 = String Subset(string=w848, offset (0)=3) -> (substring=w849:string)  [unwired: 1 in]
                                n228 = Hexadecimal String To Number(string=w849) -> (number=w847:u32)  [unwired: 2 in, 1 out]
                                n229 = local write "D (Rate) IstWert"(w847) -> ()
                                n230 = local write "D (Rate) Sollwert"(w847) -> ()
                                }
                                frame 3 {
                                n231 = String Subset(string=w852, offset (0)=3) -> (substring=w853:string)  [unwired: 1 in]
                                n232 = Hexadecimal String To Number(string=w853) -> (number=w851:u32)  [unwired: 2 in, 1 out]
                                n233 = local write "% LOW Istwert"(w851) -> ()
                                n234 = local write "% LOW Sollwert"(w851) -> ()
                                }
                                frame 4 {
                                n235 = String Subset(string=w856, offset (0)=3) -> (substring=w857:string)  [unwired: 1 in]
                                n236 = Hexadecimal String To Number(string=w857) -> (number=w855:u32)  [unwired: 2 in, 1 out]
                                n237 = local write "% HIGH Istwert"(w855) -> ()
                                n238 = local write "% High Sollwert"(w855) -> ()
                                }
                                frame 5 {
                                n239 = call "I3252_Edit_Setpoint.vi"("Read String"=w860) -> ("Setpoint is"=w859:dbl)
                                n240 = local write "SP 1 is (°C)"(w859) -> ()
                                }
                              }
                            }
                          }
                        }
                      }
                      frame #2 {
                        n241 = property on="RAM" class="Bool (strict)"("Blinking"=FALSE) -> ()  [unwired: 2 in, 2 out]
                      }
                    }
                    n242 = Not(x="RAM") -> (.not. x?=w795:bool)
                  }
                  event "Set Gauge to Zero": Value Change {
                    n243 = event-data() -> ()  [unwired: 1 in, 1 out]
                    n244 = flat-sequence {
                      tunnel: w866 -> [w871]
                      tunnel: [w871] -> w865
                      tunnel: w865 -> [w873]
                      tunnel: [w877] -> w864
                      tunnel: [w876] -> w863
                      tunnel: [w873] -> w862
                      tunnel: w864 -> [w883]
                      tunnel: w863 -> [w882]
                      tunnel: w862 -> [w878]
                      frame #0 {
                        n245 = property on="Set Gauge to Zero" class="Bool"("Blinking"=TRUE) -> ()  [unwired: 2 in, 2 out]
                      }
                      frame #1 {
                        w874 = 0 items=["sensor 1", "sensor 2", "test"] ("Sensor Nr.:")
                        n246 = call "DUAL GAUGE-Get Pressure,Status.vi"("Sensor Nr.:"=w874, "Referenz in"=w873) -> ("Pressure"=w877:dbl)  [unwired: 6 in, 3 out]
                        n247 = call "DUAL GAUGE-Offset display.vi"("W/R"=FALSE, "Referenz in"=w873) -> ("Sensor 1 Get"=w876:dbl)  [unwired: 6 in, 3 out]
                      }
                      frame #2 {
                        n248 = Add(x=w883, y=w882) -> (x+y=w879:dbl)
                        n249 = call "DUAL GAUGE-Offset display.vi"("W/R"=TRUE, "Sensor 1 Set"=w879, "Referenz in"=w878) -> ("Sensor 1 Get"=→"Current Offset (mbar)":dbl)  [unwired: 5 in, 3 out]
                      }
                      frame #3 {
                        n250 = property on="Set Gauge to Zero" class="Bool"("Blinking"=TRUE) -> ()  [unwired: 2 in, 2 out]
                      }
                    }
                    n251 = Unbundle(w870) -> ("VISA resource name out"=w869:refnum<visa-resource-name>, "error out"=w868:errorcluster)  [unwired: 2 out]
                  }
                  event "Write to File": Value Change {
                    n252 = event-data() -> ("NewVal"=w889:bool)  [unwired: 1 in]
                    n253 = local read "File Path"() -> (w885:path)
                    n254 = case shown="True" w889 {
                      tunnel: w885 -> [_ w897]
                      tunnel: "User" -> [_ w896]
                      tunnel: "Sample" -> [_ w895]
                      tunnel: [path "" ("File Path") w894] -> w886
                      frame False {
                      }
                      frame True {
                        n255 = call "Header.vi"("Sample"=w895, "User"=w896, "File Path"=w897) -> ("File Path"=w894:path)
                      }
                    }
                    n256 = Unbundle(w892) -> ("VISA resource name out"=w891:refnum<visa-resource-name>, "error out"=w890:errorcluster)  [unwired: 2 out]
                    n257 = local write "File Path"(w886) -> ()
                  }
                  event "Ramp": Value Change {
                    n258 = event-data() -> ()  [unwired: 1 in, 6 out]
                    n259 = stacked-sequence {
                      tunnel: [_ w905 _ _] -> w898
                      tunnel: [_ w904 _ _] -> w899
                      tunnel: w900 -> [_ w903 w954 _]
                      frame #0 {
                        n260 = property on="Ramp" class="Bool (strict)"("Blinking"=TRUE) -> ()  [unwired: 2 in, 2 out]
                      }
                      frame #1 {
                        n261 = for {
                          N: 6 -> [_]
                          tunnel: [w911] -> w905
                          tunnel: [w910] -> w904
                          tunnel: w903 -> [w909]
                          i -> [w907]
                          n262 = flat-sequence {
                            tunnel: w907 -> [w913]
                            tunnel: [w912] -> w908
                            tunnel: [w946] -> w911
                            tunnel: [w947] -> w910
                            tunnel: w909 -> [w948]
                            tunnel: w908 -> [w945]
                            frame #0 {
                              n263 = case shown="5" w913 {
                                tunnel: ["*D03" w917 w919 w931 "*E03" ("string") "*Z02" ("string")] -> w912
                                frame 0, Default {
                                }
                                frame 1 {
                                n264 = local read "Ramp"() -> (w915:bool)
                                n265 = Select(t="*W0D78", s=w915, f="*W0D60") -> (s? t:f=w917:string)
                                }
                                frame 2 {
                                n266 = local read "Ramp"() -> (w920:bool)
                                n267 = case shown="True" w920 {
                                tunnel: ["*W0E0000" ("string") w922] -> w919
                                frame False {
                                }
                                frame True {
                                n268 = Multiply(x="Hours", y=100.0) -> (x*y=w928:dbl)
                                n269 = Add(x=w928, y="Minutes") -> (x+y=w925:dbl)
                                n270 = Number To Hexadecimal String(1:i16 4 ("width (-)"), 2:w925) -> (0:w926:string)
                                n271 = Concatenate Strings("*W0E" ("string"), w926) -> (w922:string)
                                }
                                }
                                }
                                frame 3 {
                                n272 = local read "Ramp"() -> (w932:bool)
                                n273 = case shown="True" w932 {
                                tunnel: ["*W1E0000" ("string") w934] -> w931
                                frame False {
                                }
                                frame True {
                                n274 = Multiply(x="Soak Hours", y=100.0) -> (x*y=w940:dbl)
                                n275 = Add(x=w940, y="Soak Minutes") -> (x+y=w937:dbl)
                                n276 = Number To Hexadecimal String(1:i16 4 ("width (-)"), 2:w937) -> (0:w938:string)
                                n277 = Concatenate Strings("*W1E" ("string"), w938) -> (w934:string)
                                }
                                }
                                }
                                frame 4 {
                                }
                                frame 5 {
                                }
                              }
                            }
                            frame #1 {
                              n278 = Unbundle(w948) -> ("VISA resource name out"=w949:refnum<visa-resource-name>, "error out"=w951:errorcluster, "Delay (ms)"=w950:u32, "Write/\nRead"=w952:bool)
                              n279 = call "I3252_Comm_Interface.vi"("VISA resource name in"=w949, "error in"=w951, "Delay (ms)"=w950, "Write"=w952, "String to Write"=w945, "Read"=w952) -> ("VISA resource name out"=w947:refnum<visa-resource-name>, "error out"=w946:errorcluster)  [unwired: 2 in, 1 out]
                            }
                          }
                          n280 = Wait (ms)(milliseconds to wait=u32 1000) -> ()  [unwired: 1 out]
                        }
                      }
                      frame #2 {
                        n281 = local read "Ramp"() -> (w953:bool)
                        n282 = case shown="True" w953 {
                          tunnel: w954 -> [_ w955]
                          frame False {
                          }
                          frame True {
                            n283 = Multiply(x=10.0, y="Setpoint") -> (x*y=w960:dbl)
                            n284 = Number To Hexadecimal String(1:i16 5 ("width (-)"), 2:w960) -> (0:w961:string)
                            n285 = Concatenate Strings("*P012", w961) -> (w957:string)
                            n286 = Wait (ms)(milliseconds to wait=u32 4000) -> ()  [unwired: 1 out]
                            n287 = Unbundle(w955) -> ("VISA resource name out"=w963:refnum<visa-resource-name>, "error out"=w965:errorcluster, "Delay (ms)"=w964:u32, "Write/\nRead"=w966:bool)
                            n288 = call "I3252_Comm_Interface.vi"("VISA resource name in"=w963, "error in"=w965, "Delay (ms)"=w964, "Write"=w966, "String to Write"=w957, "Read"=w966) -> ()  [unwired: 2 in, 3 out]
                          }
                        }
                      }
                      frame #3 {
                        n289 = property on="Ramp" class="Bool (strict)"("Blinking"=FALSE) -> ()  [unwired: 2 in, 2 out]
                      }
                    }
                  }
                  event "Get SetPoint": Value Change {
                    n290 = event-data() -> ()  [unwired: 1 in, 6 out]
                    n291 = Unbundle(w972) -> ("VISA resource name out"=w976:refnum<visa-resource-name>, "error out"=w978:errorcluster, "Delay (ms)"=w977:u32, "Write/\nRead"=w979:bool)
                    n292 = call "I3252_Comm_Interface.vi"("VISA resource name in"=w976, "error in"=w978, "Delay (ms)"=w977, "Write"=w979, "String to Write"="*G01", "Read"=w979) -> ("VISA resource name out"=w971:refnum<visa-resource-name>, "error out"=w970:errorcluster, "Read String"=w975:string)  [unwired: 2 in]
                    n293 = call "I3252_Edit_Setpoint.vi"("Read String"=w975) -> ("Setpoint is"=→"Get Actual Set Point":dbl)
                  }
                }
              }
              n294 = Bundle(cluster=w391, "VISA resource name out"=w390, "error out"=w389) -> (w388:T7)  [unwired: 2 in]
            }
            frame #2 {
            }
            frame #3 {
              (unwired) "Daniel Schuster (geb. 20.03.1988)"
              n295 = node-c288(w1032) -> (w1041:T3)  [unwired: 2 in]
              n296 = node-c288(w1047) -> (w1050:T3)  [unwired: 2 in]
              n297 = node-c288(w1037) -> (w1039:T3)  [unwired: 2 in]
              n298 = node-c288(w1046) -> (w1054:T3)  [unwired: 2 in]
              n299 = timed-sequence {
                timing: w1041 -> [_]
                timing-out: [_] -> w1040
                tunnel: w1016 -> [w1097]
                tunnel: w1015 -> [w1093]
                tunnel: [w1096] -> w1008
                tunnel: w1007 -> [w1095]
                tunnel: w1006 -> [w1094]
                tunnel: [w1092] -> w1005
                tunnel: [w1091] -> w1004
                tunnel: [w1090] -> w1002
                n300 = timed-flat-sequence {
                  tunnel: w1097 -> [w1106]
                  tunnel: [w1105] -> w1096
                  tunnel: w1095 -> [w1104]
                  tunnel: w1094 -> [w1103]
                  tunnel: w1093 -> [w1102]
                  tunnel: [w1100] -> w1092
                  tunnel: [w1099] -> w1091
                  tunnel: [w1098] -> w1090
                  n301 = node-c288() -> ()  [unwired: 1 in, 1 out]
                  n302 = case shown="True" "ON (TPG 2)" {
                    tunnel: w1102 -> [w1111 w1117]
                    tunnel: w1103 -> [w1110 w1116]
                    tunnel: [w1109 w1115] -> w1099
                    tunnel: [w1108 w1114] -> w1098
                    frame False {
                      w1112 = 0.0 ("Pressure")
                      n303 = property on="ON (TPG 2)" class="Bool (strict)"("Blinking"=FALSE) -> ()  [unwired: 2 in, 2 out]
                      n304 = Bundle("Pressure"=w1112, "Pressure"=w1112) -> (w1109:cluster{"Pressure":dbl, "Pressure":dbl})  [unwired: 1 in]
                      n305 = Bundle("TPG 2 COM"=w1111, "error out"=w1110) -> (w1108:T9)  [unwired: 1 in]
                    }
                    frame True {
                      n306 = stacked-sequence {
                        tunnel: w1117 -> [_ w1130]
                        tunnel: [_ w1126] -> w1115
                        tunnel: [_ w1122] -> w1114
                        tunnel: w1116 -> [_ w1119]
                        frame #0 {
                          n307 = property on="ON (TPG 2)" class="Bool (strict)"("Blinking"=TRUE) -> ()  [unwired: 2 in, 2 out]
                        }
                        frame #1 {
                          n308 = call "PresureGetSubVI.vi"("COM in"=w1130, "Fehler (Eingang)"=w1119) -> ("Status Gauge#1"=→"Status Gauge 2#1":i32, "Status Gauge#2"=→"Status Gauge 2#2":i32, "COM out"=w1123:refnum<visa-resource-name>, "Pressure Gauge#1"=w1124:dbl, "Pressure Gauge#2"=w1127:dbl, "Cluster (Ausgang)"=w1120:errorcluster)  [unwired: 12 in]
                          "Pressure Gauge 2#1" <- w1124
                          "Pressure Gauge 2#2" <- w1127
                          n309 = Bundle("COM out"=w1123, "Cluster (Ausgang)"=w1120) -> (w1122:T10)  [unwired: 1 in]
                          n310 = Unbundle(w1120) -> ("status"=w1121:bool, "code"=w1125:i32)  [unwired: 1 out]
                          n311 = Bundle("status"=w1121, "code"=w1125) -> ()  [unwired: 1 in, 1 out]
                          n312 = Bundle("Pressure Gauge#1"=w1124, "Pressure Gauge#2"=w1127) -> (w1126:T11)  [unwired: 1 in]
                        }
                      }
                    }
                  }
                  n313 = case shown="True" "ON (TPG 1)" {
                    tunnel: w1106 -> [w1134 w1140]
                    tunnel: [w1133 w1139] -> w1105
                    tunnel: w1104 -> [w1132 w1138]
                    tunnel: [w1131 w1137] -> w1100
                    frame False {
                      w1135 = 0.0 ("Pressure")
                      n314 = property on="ON (TPG 1)" class="Bool (strict)"("Blinking"=FALSE) -> ()  [unwired: 2 in, 2 out]
                      n315 = Bundle("Pressure"=w1135, "Pressure"=w1135) -> (w1131:cluster{"Pressure":dbl, "Pressure":dbl})  [unwired: 1 in]
                      n316 = Bundle("TPG 1 COM"=w1134, "error out"=w1132) -> (w1133:T12)  [unwired: 1 in]
                    }
                    frame True {
                      n317 = stacked-sequence {
                        tunnel: w1140 -> [_ w1153]
                        tunnel: [_ w1146] -> w1139
                        tunnel: w1138 -> [_ w1143]
                        tunnel: [_ w1142] -> w1137
                        frame #0 {
                          n318 = property on="ON (TPG 1)" class="Bool (strict)"("Blinking"=TRUE) -> ()  [unwired: 2 in, 2 out]
                        }
                        frame #1 {
                          n319 = call "PresureGetSubVI.vi"("COM in"=w1153, "Fehler (Eingang)"=w1143) -> ("Status Gauge#1"=→"Status Gauge 1#1":i32, "Status Gauge#2"=→"Status Gauge 1#2":i32, "COM out"=w1147:refnum<visa-resource-name>, "Pressure Gauge#1"=w1148:dbl, "Pressure Gauge#2"=w1150:dbl, "Cluster (Ausgang)"=w1144:errorcluster)  [unwired: 12 in]
                          "Pressure Gauge 1#1" <- w1148
                          "Pressure Gauge 1#2" <- w1150
                          n320 = Bundle("COM out"=w1147, "Cluster (Ausgang)"=w1144) -> (w1146:T10)  [unwired: 1 in]
                          n321 = Unbundle(w1144) -> ("status"=w1145:bool, "code"=w1149:i32)  [unwired: 1 out]
                          n322 = Bundle("status"=w1145, "code"=w1149) -> ()  [unwired: 1 in, 1 out]
                          n323 = Bundle("Pressure Gauge#1"=w1148, "Pressure Gauge#2"=w1150) -> (w1142:T11)  [unwired: 1 in]
                        }
                      }
                    }
                  }
                  n324 = node-c288() -> ()  [unwired: 1 in, 1 out]
                }
              }
              n325 = timed-sequence {
                timing: w1050 -> [_]
                timing-out: [_] -> w1049
                tunnel: w1048 -> [w1163]
                tunnel: [w1162] -> w1043
                tunnel: [w1161] -> w1042
                tunnel: [w1160] -> w1029
                n326 = timed-flat-sequence {
                  tunnel: w1163 -> [w1167]
                  tunnel: [w1166] -> w1162
                  tunnel: [w1165] -> w1161
                  tunnel: [w1164] -> w1160
                  n327 = node-c288() -> ()  [unwired: 1 in, 1 out]
                  n328 = case shown="True" "ON" {
                    tunnel: w1167 -> [w1171 w1176]
                    tunnel: [w1170 w1175] -> w1166
                    tunnel: [w1169 w1174] -> w1165
                    tunnel: [_ w1173] -> w1164
                    frame False {
                      n329 = Unbundle(w1171) -> ("VISA resource name out"=w1170:refnum<visa-resource-name>, "error out"=w1169:errorcluster)  [unwired: 2 out]
                      n330 = property on="ON" class="Bool (strict)"("Blinking"=FALSE) -> ()  [unwired: 2 in, 2 out]
                    }
                    frame True {
                      n331 = stacked-sequence {
                        tunnel: w1176 -> [_ w1181]
                        tunnel: [_ w1180] -> w1175
                        tunnel: [_ w1179] -> w1174
                        tunnel: [_ w1178] -> w1173
                        frame #0 {
                          n332 = property on="ON" class="Bool (strict)"("Blinking"=TRUE) -> ()  [unwired: 2 in, 2 out]
                        }
                        frame #1 {
                          n333 = Unbundle(w1181) -> ("VISA resource name out"=w1185:refnum<visa-resource-name>, "error out"=w1183:errorcluster, "Delay (ms)"=w1184:u32, "Write/\nRead"=w1182:bool)
                          n334 = call "I3252_Comm_Interface.vi"("VISA resource name in"=w1185, "error in"=w1183, "Delay (ms)"=w1184, "Write"=w1182, "String to Write"="*V01", "Read"=w1182) -> ("VISA resource name out"=w1180:refnum<visa-resource-name>, "error out"=w1179:errorcluster, "Read String"=w1178:string)  [unwired: 2 in]
                        }
                      }
                    }
                  }
                  n335 = node-c288() -> ()  [unwired: 1 in, 1 out]
                }
              }
              n336 = timed-sequence {
                timing: w1039 -> [_]
                timing-out: [_] -> w1038
                tunnel: w1036 -> [w1059]
                tunnel: w1035 -> [w1058]
                tunnel: [w1057] -> w1033
                tunnel: [w1056] -> w1034
                tunnel: [w1055] -> w1030
                n337 = timed-flat-sequence {
                  tunnel: w1059 -> [w1064]
                  tunnel: w1058 -> [w1063]
                  tunnel: [w1062] -> w1057
                  tunnel: [w1061] -> w1056
                  tunnel: [w1060] -> w1055
                  n338 = node-c288() -> ()  [unwired: 1 in, 1 out]
                  n339 = case shown="False" "ON" {
                    tunnel: w1064 -> [w1068 w1074]
                    tunnel: w1063 -> [w1069 w1073]
                    tunnel: [w1068 w1072] -> w1062
                    tunnel: [w1069 w1071] -> w1061
                    tunnel: [0.0 ("Reading") w1070] -> w1060
                    frame False {
                      n340 = property on="ON" class="Bool (strict)"("Blinking"=FALSE) -> ()  [unwired: 2 in, 2 out]
                    }
                    frame True {
                      n341 = stacked-sequence {
                        tunnel: w1074 -> [_ w1081]
                        tunnel: w1073 -> [_ w1080]
                        tunnel: [_ w1079] -> w1072
                        tunnel: [_ w1078] -> w1071
                        tunnel: [_ w1076] -> w1070
                        frame #0 {
                          n342 = property on="ON" class="Bool (strict)"("Blinking"=TRUE) -> ()  [unwired: 2 in, 2 out]
                        }
                        frame #1 {
                          n343 = call "VC840_Read.vi"("error in (no error)"=w1080, "VISA resource name"=w1081) -> ("error out"=w1078:errorcluster, "Unit"=→"Unit 2":string, "Reading"=w1076:dbl, "VISA resource name out"=w1079:refnum<visa-resource-name>, "Status"=→"Status 2":T2, "Mode"=→"Mode 2":enum16{"?", "Diode", "Beep", "DC", "AC"})  [unwired: 4 out]
                          "Reading 2" <- w1076
                        }
                      }
                    }
                  }
                  n344 = node-c288() -> ()  [unwired: 1 in, 1 out]
                }
              }
              n345 = timed-sequence {
                timing: w1054 -> [_]
                timing-out: [_] -> w1053
                tunnel: w1052 -> [w1197]
                tunnel: w1051 -> [w1196]
                tunnel: [w1195] -> w1045
                tunnel: [w1194] -> w1044
                tunnel: [w1193] -> w1031
                n346 = timed-flat-sequence {
                  tunnel: w1197 -> [w1202]
                  tunnel: w1196 -> [w1201]
                  tunnel: [w1200] -> w1195
                  tunnel: [w1199] -> w1194
                  tunnel: [w1198] -> w1193
                  n347 = node-c288() -> ()  [unwired: 1 in, 1 out]
                  n348 = case shown="True" "ON" {
                    tunnel: w1202 -> [w1206 w1212]
                    tunnel: w1201 -> [w1207 w1211]
                    tunnel: [w1206 w1210] -> w1200
                    tunnel: [w1207 w1209] -> w1199
                    tunnel: [0.0 ("Reading") w1208] -> w1198
                    frame False {
                      n349 = property on="ON" class="Bool (strict)"("Blinking"=FALSE) -> ()  [unwired: 2 in, 2 out]
                    }
                    frame True {
                      n350 = stacked-sequence {
                        tunnel: w1212 -> [_ w1219]
                        tunnel: w1211 -> [_ w1218]
                        tunnel: [_ w1217] -> w1210
                        tunnel: [_ w1216] -> w1209
                        tunnel: [_ w1214] -> w1208
                        frame #0 {
                          n351 = property on="ON" class="Bool (strict)"("Blinking"=TRUE) -> ()  [unwired: 2 in, 2 out]
                        }
                        frame #1 {
                          n352 = call "VC840_Read.vi"("error in (no error)"=w1218, "VISA resource name"=w1219) -> ("error out"=w1216:errorcluster, "Unit"=→"Unit 1":string, "Reading"=w1214:dbl, "VISA resource name out"=w1217:refnum<visa-resource-name>, "Status"=→"Status 1":T2, "Mode"=→"Mode 1":enum16{"?", "Diode", "Beep", "DC", "AC"})  [unwired: 4 out]
                          "Reading 1" <- w1214
                        }
                      }
                    }
                  }
                  n353 = node-c288() -> ()  [unwired: 1 in, 1 out]
                }
              }
              n354 = Tick Count (ms)() -> (millisecond timer value=w1017:u32)
              n355 = Subtract(x=w1017, y=w1022) -> (x-y=w1021:u32)
              n356 = Divide(x=w1021, y=u32 1000) -> (x/y=w1019:dbl)
              n357 = node-c288(w1053) -> ()  [unwired: 1 out]
              n358 = node-c288(w1038) -> ()  [unwired: 1 out]
              n359 = node-c288(w1049) -> ()  [unwired: 1 out]
              n360 = To Double Precision Float(number=w1019) -> (double precision float=w1023:dbl)
              "current time (s)" <- w1023
              n361 = node-c288(w1040) -> ()  [unwired: 1 out]
              n362 = Unbundle(w1004) -> ("Pressure Gauge#1"=w1003:dbl, "Pressure Gauge#2"=w1001:dbl)
              "Pressure OpenPort2" <- w1001
              "Pressure Pirani 2" <- w1003
              n363 = Unbundle(w1005) -> ("Pressure Gauge#1"=w1014:dbl, "Pressure Gauge#2"=w1009:dbl)
              "Pressure Baratron 2" <- w1014
              "Pressure FullRange 2" <- w1009
            }
            frame #4 {
              n364 = Build Array (concatenate)(w1239, w1243) -> (w1238:dbl[])
              n365 = Build Array (concatenate)(w1242, w1244) -> (w1237:dbl[])
              n366 = Build Array (concatenate)(w1240, w1231) -> (w1235:dbl[])
              n367 = Build Array (concatenate)(w1241, w1232) -> (w1236:dbl[])
              n368 = Greater?(x=w1263, y="Pressure Limit (mbar)") -> (0:w1266:bool)
              n369 = case shown="False" w1266 {
                frame False {
                  n370 = property on="Standby" class="Bool (strict)"("DisabledEnum"=T6."Enabled" ("Disabled")) -> ()  [unwired: 2 in, 2 out]
                }
                frame True {
                  n371 = property on="Standby" class="Bool (strict)"("Val(Sgnl)"=TRUE ("Standby"), "DisabledEnum"=T6."Disabled" ("Disabled")) -> ()  [unwired: 2 in, 2 out]
                }
              }
              n372 = call "Resistivity_Calculation.vi"("Reading 1 (V)"=w1256, "Constant"="4PP constant", "Thickness (nm)"="Thickness (nm)", "Reading 2 (A)"=w1264) -> ("Resivtivity (Ohm*cm)"=w1248:dbl, "Current"=w1249:dbl, "Voltage"=w1250:dbl)
              "Resistivity (Ohm*cm)" <- w1248
              "Voltage (V)" <- w1250
              "Current (A)" <- w1249
              n373 = call "I3252_Edit_Temperature.vi"("Temp. String"=w1265) -> ("Temp. (°C)"=w1259:dbl)
              "(°C)" <- w1259
              n374 = Build Array (concatenate)(w1261, w1262) -> (w1258:dbl[])
              n375 = Build Array (concatenate)(w1260, w1259) -> (w1246:dbl[])
              n376 = Build Array (concatenate)(w1257, w1250) -> (w1255:dbl[])
              n377 = Build Array (concatenate)(w1254, w1249) -> (w1252:dbl[])
              n378 = Build Array (concatenate)(w1253, w1248) -> (w1251:dbl[])
              n379 = Build Array(w1250, w1249, w1248) -> (w1247:dbl[])
            }
            frame #5 {
              n380 = Bundle(w1297, w1296) -> (w1281:cluster{dbl[], dbl[]})  [unwired: 1 in]
              n381 = Bundle(w1297, w1295) -> (w1280:cluster{dbl[], dbl[]})  [unwired: 1 in]
              n382 = Bundle(w1297, w1294) -> (→"Pirani (VVP1 Scroll)":cluster{dbl[], dbl[]})  [unwired: 1 in]
              n383 = Bundle(w1297, w1293) -> (→"Pressure OpenPort":cluster{dbl[], dbl[]})  [unwired: 1 in]
              n384 = Bundle(w1297, w1301) -> (→"Thermocouple (Sample holder 1)":cluster{dbl[], dbl[]})  [unwired: 1 in]
              n385 = Bundle(w1297, w1303) -> (→"Voltage":cluster{dbl[], dbl[]})  [unwired: 1 in]
              n386 = Bundle(w1297, w1304) -> (→"Current":cluster{dbl[], dbl[]})  [unwired: 1 in]
              n387 = Bundle(w1297, w1305) -> (→"Resistivity":cluster{dbl[], dbl[]})  [unwired: 1 in]
              n388 = Build Array(w1281, w1280) -> (→"TPG 1":cluster{dbl[], dbl[]}[])
              n389 = Build Array (concatenate)(w1300, w1310, w1309, w1299, w1288, w1284, w1282) -> (w1317:dbl[])
              "appended array" <- w1317
            }
            frame #6 {
              n390 = Unbundle(w1327) -> ("COM out"=w1326:refnum<visa-resource-name>, "Cluster (Ausgang)"=w1325:errorcluster)
              n391 = Unbundle(w1324) -> ("COM out"=w1323:refnum<visa-resource-name>, "Cluster (Ausgang)"=w1322:errorcluster)
              n392 = call "Elapsed Time"("Time Target (s)"="Intervall (s)") -> ("Time has Elapsed"=w1320:bool)  [unwired: 11 in, 7 out]
              n393 = And(x="Write to File", y=w1320) -> (x .and. y?=w1318:bool)
              n394 = case shown="True" w1318 {
                tunnel: [w1349 w1355] -> w1341
                tunnel: "File Path" -> [w1349 w1353]
                tunnel: w1334 -> [_ w1351]
                frame False {
                  n395 = property on="Write to File" class="Bool (strict)"("Blinking"=FALSE) -> ()  [unwired: 2 in, 2 out]
                }
                frame True {
                  n396 = flat-sequence {
                    tunnel: [w1357] -> w1354
                    tunnel: w1353 -> [w1357]
                    tunnel: [w1356] -> w1352
                    tunnel: w1351 -> [w1356]
                    tunnel: [w1362] -> w1355
                    tunnel: w1354 -> [w1361]
                    tunnel: w1352 -> [w1360]
                    frame #0 {
                      n397 = property on="Write to File" class="Bool (strict)"("Blinking"=TRUE) -> ()  [unwired: 2 in, 2 out]
                    }
                    frame #1 {
                      n398 = call-poly <vilib>:"Write To Spreadsheet File.vi"("format (%.3f)"="%g", "append to file? (new file:F)"=TRUE ("transpose? (no:F)"), "1D data"=w1360, "file path (dialog if empty)"=w1361) -> ("new file path (Not A Path if cancelled)"=w1362:path)  [unwired: 4 in]
                    }
                  }
                }
              }
              n399 = Merge Errors(w1345, w1344, w1342, w1325, w1322) -> (w1343:errorcluster)
              n400 = call <vilib>:"Simple Error Handler.vi"("error in (no error)"=w1343) -> ("error?"=w1328:bool)  [unwired: 4 in, 4 out]
              n401 = local write "File Path"(w1341) -> ()
            }
            frame #7 {
              w1379 = u32 1000 ("y")
              n402 = Tick Count (ms)() -> (millisecond timer value=w1381:u32)
              n403 = Subtract(x=w1381, y=w1380) -> (x-y=w1382:u32)
              n404 = VISA Flush I/O Buffer(VISA resource name=w1373, error in (no error)=w1372) -> (VISA resource name out=w1370:refnum<visa-resource-name>, error out=w1371:errorcluster)  [unwired: 1 in]
              n405 = VISA Flush I/O Buffer(VISA resource name=w1366, error in (no error)=w1365) -> (VISA resource name out=w1369:refnum<visa-resource-name>, error out=w1368:errorcluster)  [unwired: 1 in]
              n406 = Divide(x=w1382, y=w1379) -> (x/y=→"loop time (s)":dbl)
              n407 = Subtract(x=u32 1, y=u32 1) -> (x-y=w1383:u32)
              n408 = Multiply(x=w1383, y=w1379) -> (x*y=w1385:u32)
              n409 = Wait (ms)(milliseconds to wait=w1385) -> ()  [unwired: 1 out]
              n410 = Bundle("COM out"=w1370, "error out"=w1371, "COM out"=w1369, "error out"=w1368) -> (w1367:T13)  [unwired: 1 in]
            }
            frame #8 {
              n411 = Tick Count (ms)() -> (millisecond timer value=w1405:u32)
              n412 = Subtract(x=w1405, y=w1403) -> (x-y=w1404:u32)
              n413 = Divide(x=w1404, y=w1402) -> (x/y=→"data logger intervall (s)":dbl)
            }
          }
          n414 = Exclusive Or(1:"stop", 2:w154) -> (0:w155:bool)
        }
      }
      frame #4 {
        n415 = call "VC840_Close.vi"("error in (no error)"=w1424, "VISA resource name"=w1425) -> ("error out"=w1433:errorcluster)  [unwired: 9 in]
        n416 = call "VC840_Close.vi"("error in (no error)"=w1426, "VISA resource name"=w1427) -> ("error out"=w1431:errorcluster)  [unwired: 9 in]
        n417 = VISA Close(VISA resource name=w1429, error in (no error)=w1428) -> (error out=w1430:errorcluster)
        n418 = Unbundle(w1422) -> ("COM out"=w1421:refnum<visa-resource-name>, "error out"=w1420:errorcluster, "COM out"=w1418:refnum<visa-resource-name>, "error out"=w1419:errorcluster)
        n419 = VISA Close(VISA resource name=w1421, error in (no error)=w1420) -> ()  [unwired: 1 out]
        n420 = VISA Close(VISA resource name=w1418, error in (no error)=w1419) -> ()  [unwired: 1 out]
        n421 = Merge Errors(w1430, w1431, w1433) -> (w1432:errorcluster)
        n422 = call <vilib>:"Simple Error Handler.vi"("error in (no error)"=w1432) -> ("error?"=w1423:bool)  [unwired: 1 in, 7 out]
        n423 = Stop(stop? (T)=w1423) -> ()
      }
    }
  }
